vi "AbelFcsMain.vi"() -> ()   [LabVIEW 2011]
uses:
  Camera/vi/ccdChipPixels.vi
  Camera/vi/GlobalSetGetConfigureCamera.vi
  Camera/lib/System Files/user.lib/atmcd32d.llb/Shutter_mode typedef.ctl
  Camera/lib/System Files/user.lib/atmcd32d.llb/Shutter_type typedef.ctl
  Variables/GetPicture.vi
  Camera/vi/StopGetPic.vi
  Camera/vi/CamDef.vi
  Variables/GlobalLaserInterface.vi
  Variables/patternImg.vi
  <vilib>/vision/Image Controls.llb/IMAQ Rounding Mode.ctl
  Variables/GlobalConAxisPI.vi
  Variables/GlobalCameraHandle.vi
  <vilib>/vision/Pattern Matching.llb/IMAQ Match Range Setting.ctl
  <vilib>/vision/Pattern Matching.llb/IMAQ Curve Parameters.ctl
panel:
  out "subarray":dbl[](array[numeric])
  in  "Settings (GeometricMatching)":T3={"Curve Parameters"={"Extraction Mode"=0, "Edge Threshold"=75, "Edge Filter Size"=1, "Min Length"=25, "Row Search Step Size"=15, "Col Search Step Size"=15, "Max Endpoint Gap"=10, "Closed"=FALSE, "Subpixel"=FALSE}, "Match Mode"={"Rotation"=TRUE, "Scale"=FALSE, "Occlusion"=TRUE, "Reserved"=FALSE, "Reserved"=FALSE, "Reserved"=FALSE}, "Range Settings"=[{"Match Constraints"=0, "Min"=0.0, "Max"=360.0}, {"Match Constraints"=2, "Min"=0.0, "Max"=25.0}], "Number of Matches"=5, "Minimum Match Score"=600.0, "SubPixel Accuracy"=FALSE, "Adv. Geometric Match Options 2"=[{"Setup Data Item"=21, "Item Value"=0.0}, {"Setup Data Item"=22, "Item Value"=1.0}]} {"Curve Parameters"."Extraction Mode" items=["Normal", "Uniform Regions"]; "Curve Parameters"."Edge Filter Size" items=["Fine", "Normal", "Contour Tracing"]; "Curve Parameters"."Max Endpoint Gap" min=0; "Curve Parameters"."Col Search Step Size" min=1 max=255 step=1; "Curve Parameters"."Row Search Step Size" min=1 max=255 step=1; "Curve Parameters"."Min Length" min=0; "Curve Parameters"."Edge Threshold" min=1 max=350 step=1; "Range Settings"."Max" format="%.2f"; "Range Settings"."Min" format="%.2f"; "Range Settings"."Match Constraints" items=["Rotation Angle (degrees)", "Scale Factor (%)", "Occlusion (%)"]; "Adv. Geometric Match Options 2"."Setup Data Item" items=["Curve Extraction Mode", "Curve Edge Threshold", "Curve Edge Filter Size", "Min Curve Length", "Curve Row Search Step Size", "Curve Col Search Step Size", "Curve Max Endpoint Gap", "Extract Closed Curves", "Enable Subpixel Curve Extraction", "Enable Correlation Score", "Enable Subpixel Accuracy", "Subpixel Iterations", "Subpixel Tolerance", "Initial Match List Length", "Enable Target Template Curve Score", "Min Match Separation Distance", "Min Match Separation Angle", "Min Match Separation Scale", "Max Match Overlap", "Enable Coarse Result", "Enable Calibration Support", "Enable Contrast Reversal", "Search Strategy", "Refinement Match Factor", "Subpixel Match Factor"]}
  in  "Tab Control":T4(tab)
  out "Histogram":i32[][](graph)
  out "Trace":i32[][](graph)=[[2, 0, 0, 1, 1, 1, 0, 0, 0, 1, 0, 1, 0, 1, 2, 2, 0, 3, 0, 2, 2, 1, 3, 1, 0, 1, 1, 1, 0, 1, 3, 1, 0, 2, 0, 1, 0, 1, 1, 0, 1, 1, 3, 1, 0, 2, 0, 1, 1, 0, 0, 2, 0, 0, 1, 1, 1, 0, 0, 1, 0, 1, 0, 0, 0, 1, 2, 1, 1, 2, 0, 2, 4, 3, 1, 1, 0, 0, 1, 1, 2, 0, 1, 1, 0, 0, 0, 1, 1, 1, 1, 3, 0, 0, 1, 0, 0, 0, 2, 1, 1, 1, 2, 1, 0, 1, 1, 0, 0, 2, 1, 1, 0, 0, 1, 1, 1, 1, 0, 2, 2, 0, 1, 2, 1, 0, 3, 0, 2, 1, 3, 0, 1, 1, 0, 0, 3, 0, 0, 0, 0, 0, 0, 0, 0, 0, 0, 0, 0, 0, 0, 0, 0, 0, 0, 0, 0, 0, 0, 0, 0, 0, 0, 0, 0, 0, 0, 0, 0, 0, 0, 0, 0, 0, 0, 0, 0, 0, 0, 0, 0, 0, 0, 0, 0, 0, 0, 0, 0, 0, 0, 0, 0, 0, 0, 0, 0, 0, 0, 0], [1, 2, 2, 0, 0, 0, 1, 2, 1, 2, 1, 1, 1, 0, 0, 0, 3, 1, 0, 1, 0, 2, 0, 2, 1, 1, 0, 0, 1, 0, 1, 2, 1, 0, 0, 0, 0, 0, 1, 0, 1, 0, 2, 0, 1, 0, 0, 0, 0, 1, 1, 3, 0, 0, 0, 2, 0, 0, 2, 0, 1, 1, 0, 0, 2, 0, 2, 1, 0, 1, 1, 0, 1, 1, 0, 0, 0, 1, 0, 0, 1, 0, 0, 0, 0, 1, 0, 1, 1, 1, 1, 0, 0, 0, 1, 1, 1, 0, 1, 0, 0, 0, 1, 1, 1, 0, 0, 1, 1, 3, 1, 0, 0, 0, 0, 0, 0, 0, 1, 2, 1, 0, 0, 0, 2, 3, 3, 2, 0, 1, 1, 1, 0, 0, 4, 0, 1, 2, 0, 0, 0, 2, 0, 0, 0, 0, 0, 0, 0, 0, 0, 0, 0, 0, 0, 0, 0, 0, 0, 0, 0, 0, 0, 0, 0, 0, 0, 0, 0, 0, 0, 0, 0, 0, 0, 0, 0, 0, 0, 0, 0, 0, 0, 0, 0, 0, 0, 0, 0, 0, 0, 0, 0, 0, 0, 0, 0, 0, 0, 0], [2, 2, 0, 1, 2, 0, 1, 0, 2, 3, 1, 0, 1, 0, 1, 0, 0, 0, 0, 2, 1, 0, 0, 2, 2, 0, 0, 0, 3, 0, 0, 2, 2, 2, 0, 3, 0, 3, 1, 3, 1, 3, 1, 0, 3, 1, 3, 3, 1, 1, 1, 1, 2, 0, 1, 0, 1, 1, 1, 3, 0, 2, 3, 1, 1, 1, 0, 1, 0, 1, 2, 3, 1, 2, 1, 3, 0, 2, 0, 2, 0, 1, 0, 2, 2, 1, 1, 3, 1, 2, 1, 1, 1, 3, 0, 0, 0, 0, 1, 1, 1, 0, 1, 0, 2, 1, 1, 0, 1, 0, 1, 2, 2, 2, 2, 0, 1, 0, 0, 0, 1, 1, 2, 0, 0, 1, 5, 2, 2, 0, 2, 0, 2, 2, 2, 0, 1, 0, 6, 0, 0, 0, 0, 0, 0, 0, 0, 0, 0, 0, 0, 0, 0, 0, 0, 0, 0, 0, 0, 0, 0, 0, 0, 0, 0, 0, 0, 0, 0, 0, 0, 0, 0, 0, 0, 0, 0, 0, 0, 0, 0, 0, 0, 0, 0, 0, 0, 0, 0, 0, 0, 0, 0, 0, 0, 0, 0, 0, 0, 0], [0, 0, 1, 0, 1, 1, 0, 0, 0, 1, 1, 0, 1, 0, 0, 0, 0, 0, 2, 0, 0, 0, 0, 2, 0, 0, 0, 1, 1, 2, 1, 1, 1, 2, 1, 0, 0, 3, 0, 1, 1, 0, 0, 0, 0, 1, 0, 0, 2, 1, 0, 0, 1, 1, 1, 2, 2, 0, 1, 0, 0, 1, 0, 1, 1, 0, 0, 2, 1, 1, 2, 1, 1, 0, 0, 0, 0, 2, 1, 0, 0, 0, 0, 1, 0, 1, 0, 0, 0, 0, 1, 0, 0, 0, 0, 1, 0, 1, 1, 1, 0, 2, 3, 1, 1, 0, 1, 1, 1, 0, 1, 0, 0, 1, 1, 0, 2, 0, 0, 0, 0, 3, 0, 0, 0, 0, 0, 0, 0, 0, 1, 0, 2, 0, 0, 0, 1, 2, 2, 0, 1, 0, 0, 0, 0, 0, 0, 0, 0, 0, 0, 0, 0, 0, 0, 0, 0, 0, 0, 0, 0, 0, 0, 0, 0, 0, 0, 0, 0, 0, 0, 0, 0, 0, 0, 0, 0, 0, 0, 0, 0, 0, 0, 0, 0, 0, 0, 0, 0, 0, 0, 0, 0, 0, 0, 0, 0, 0, 0, 0]]
  out "Point":dbl[][](graph)
  out "Image Out":T5(plugin-control)
  out "Image Number":u32
  out "acquired FPS":dbl
  out "Image":i32[][](graph)
  out "AM image":T5(plugin-control)
  out "Number of Particles":i32
  out "Image 2":dbl[][](graph)
  out "Auto Measure Points":i32
  out "NxtAutMesPoint":i32
  out "Pattern":dbl[][](array[numeric])
  out "X Steps":dbl
  out "3dAbelFcs":bool=TRUE
  out "Y Steps":dbl
  out "Z Steps":dbl
  out "concatenated string":string
  out "Global Stop":bool=TRUE
  out "Stop Measurement":bool
  in  "DeviceTabs":T6(tab)
  in  "WS File Tree":string(tree)
  out "Workspace":path=path "X:/MTusers/Christoph/2011-02-01 Andi/2011-02-01.msw"
  in  "New MSW":bool
  in  "Open MSW":bool
  in  "Sample description":string
  in  "Save Files":bool=TRUE
  out "Last Image File No":i32=-1
  in  "Get Position":bool
  in  "Move Stage":bool
  in  "X-Position":dbl=48.0021 caption="X" min=0.0 max=200.0 step=0.1 format="%1.3f um"
  in  "Y-Position":dbl=19.9997 caption="Y" min=0.0 max=200.0 step=0.1 format="%1.3f um"
  in  "Z-Position":dbl=69.999 caption="Z" min=0.0 max=200.0 step=0.1 format="%1.3f um"
  out "x-position":dbl format="%.3f"
  out "y-position":dbl format="%.3f"
  out "z-position":dbl format="%.3f"
  in  "CFD Settings":T7={"Sync Level"=17, "Sync ZeroX"=0, "Sync Offset"=0, "Chan Settings"=[{"CHx Level"=50, "CHx ZeroX"=10, "CHx Offset"=-22150}, {"CHx Level"=50, "CHx ZeroX"=10, "CHx Offset"=-21850}, {"CHx Level"=75, "CHx ZeroX"=10, "CHx Offset"=-6000}, {"CHx Level"=75, "CHx ZeroX"=10, "CHx Offset"=-5700}]}
  in  "Laser  Profile":string="1"
  in  "Auto Exposure::Mode":u32(ring) items=["Relative"=0, "Ignored"=5]
  in  "Brightness::Mode":u32(ring) items=["Relative"=0, "Ignored"=5]
  in  "Gain::Mode":u32(ring) items=["Absolute"=1, "Auto"=3, "Relative"=0, "Ignored"=5]
  in  "Gamma::Mode":u32(ring)=2 items=["Relative"=0, "Off"=2, "Ignored"=5]
  in  "Shutter::Mode":u32(ring) items=["Auto"=3, "Relative"=0, "Ignored"=5]
  in  "Trigger::Trigger Activation":u32(ring) items=["Level Low", "Level High"]
  in  "Trigger::Trigger Mode":u32(ring)=16 items=["Mode 0"=0, "Mode 1"=1, "Mode 15"=15, "Off"=16]
  in  "Trigger Delay::Mode":u32(ring)=2 items=["Absolute"=1, "Relative"=0, "Off"=2, "Ignored"=5]
  in  "Brightness::Value":dbl=16.0 min=0.0 max=1023.0 step=1.0
  in  "Shutter::Value":dbl=436.0 min=1.0 max=4095.0 step=1.0
  in  "Auto Exposure::Value":dbl=125.0 min=50.0 max=205.0 step=1.0
  in  "Gain::Value":dbl min=0.0 max=680.0 step=1.0
  in  "Trigger::Trigger Parameter":u32 max=0
  in  "Get Temperature":bool
  in  "SET CCD":bool
  in  "OPEN SHUTER":bool
  in  "Close":bool
  in  "Gain":bool
  in  "Start":bool
  in  "Stop":bool
  in  "Exposure":bool
  in  "Set Temperature":bool
  in  "duty cycle":dbl=0.5 format="%.6f"
  in  "frequency":dbl=1.0 format="%.6f"
  in  "PI SystemNumber":i32=1
  in  "Image Measurent Parameters":T8
  in  "Measurement Tab Control":T9(tab)
  in  "SCANNER EMERGENCY":bool
  in  "Stop Program":bool
  out "Task":T10(ring)
  in  "Point Defocussed Cam":bool
  in  "Adjustment":bool
  in  "Laser pulse duration":i32[](array[numeric]) min=2 max=100000 step=1 format="%d µs"
  in  "Measurement Time":i32=60 min=10 format="%.0d s"
  in  "Point Measurement":bool
  out "Counts":u32[](array[numeric])
  in  "Axis":enum32{"x-y", "x-z", "y-x", "y-z", "z-x", "z-y"}(ring)
  in  "Picture size 2":dbl=10.0 min=0.1 max=200.0 format="%1.1f um"
  in  "Picture size":dbl=10.0 min=0.1 max=200.0 format="%1.1f um"
  in  "Pixel time":dbl=3.0 min=0.1 max=100.0 step=0.1 format="%.1f ms"
  in  "Resolution":dbl=0.08 min=0.01 max=10.0 step=0.01 format="%.2f µm"
  out "Measure. time":dbl format="%7.1f s"
  in  "Aquire Image":bool
  out "y":i16=500
  out "x":i16=500
  in  "Save Color Image":bool
  in  "Cam (Defocused)":bool
  in  "How long?":bool
  out "Estimated Time (h)":dbl
  in  "Mesaurement Time (Sec) / Step":dbl
  in  "Start 3D FCS Abel Scan":bool
  in  "FCS Point Measurement":bool
  in  "Z Stepsize":dbl
  in  "Y Stepsize":dbl
  in  "X Stepsize":dbl
  in  "Z End":dbl
  in  "Y End":dbl
  in  "X End":dbl
  in  "Z Start":dbl
  in  "Y Start":dbl
  in  "X Start":dbl
  in  "Find Mols":bool
  in  "Filter":bool=TRUE
  in  "Remove Outliers":i32=10
  in  "Exclude / Include X":bool
  in  "X Start 2":dbl
  in  "X End 2":dbl
  in  "Exclude / Include Y":bool
  in  "Y Start 2":dbl
  in  "Y End 2":dbl
  in  "Measurement Parameter 1":T11 items=["Center of Mass X", "Center of Mass Y", "First Pixel X", "First Pixel Y", "Bounding Rect Left", "Bounding Rect Top", "Bounding Rect Right", "Bounding Rect Bottom", "Max Feret Diameter Start X", "Max Feret Diameter Start Y", "Max Feret Diameter End X", "Max Feret Diameter End Y", "Max Horiz. Segment Length Left", "Max Horiz. Segment Length Right", "Max Horiz. Segment Length Row", "-", "Bounding Rect Width", "Bounding Rect Height", "Bounding Rect Diagonal", "Perimeter", "Convex Hull Perimeter", "Holes' Perimeter", "Max Feret Diameter", "Equivalent Ellipse Major Axis", "Equivalent Ellipse Minor Axis", "Equivalent Ellipse Minor Axis (Feret)", "Equivalent Rect Long Side", "Equivalent Rect Short Side", "Equivalent Rect Diagonal", "Equivalent Rect Short Side (Feret)", "Average Horiz. Segment Length", "Average Vert. Segment Length", "Hydraulic Radius", "Waddel Disk Diameter", "-", "Area", "Holes' Area", "Particle & Holes' Area", "Convex Hull Area", "Image Area", "-", "Number of Holes", "Number of Horiz. Segments", "Number of Vert. Segments", "-", "Orientation", "Max Feret Diameter Orientation", "-", "% Area/Image Area", "% Area/(Particle & Holes' Area)", "Ratio of Equivalent Ellipse Axes", "Ratio of Equivalent Rect Sides", "-", "Elongation Factor", "Compactness Factor", "Heywood Circularity Factor", "Type Factor", "-", "Sum X", "Sum Y", "Sum XX", "Sum XY", "Sum YY", "Sum XXX", "Sum XXY", "Sum XYY", "Sum YYY", "-", "Moment of Inertia XX", "Moment of Inertia XY", "Moment of Inertia YY", "Moment of Inertia XXX", "Moment of Inertia XXY", "Moment of Inertia XYY", "Moment of Inertia YYY", "Norm. Moment of Inertia XX", "Norm. Moment of Inertia XY", "Norm. Moment of Inertia YY", "Norm. Moment of Inertia XXX", "Norm. Moment of Inertia XXY", "Norm. Moment of Inertia XYY", "Norm. Moment of Inertia YYY", "Hu Moment 1", "Hu Moment 2", "Hu Moment 3", "Hu Moment 4", "Hu Moment 5", "Hu Moment 6", "Hu Moment 7"]
  in  "Range Lower Value Par 1":dbl
  in  "Range Upper Value  Par 1":dbl
  in  "Ex/In Par 1":bool
  in  "Measurement Parameter 2":T11 items=["Center of Mass X", "Center of Mass Y", "First Pixel X", "First Pixel Y", "Bounding Rect Left", "Bounding Rect Top", "Bounding Rect Right", "Bounding Rect Bottom", "Max Feret Diameter Start X", "Max Feret Diameter Start Y", "Max Feret Diameter End X", "Max Feret Diameter End Y", "Max Horiz. Segment Length Left", "Max Horiz. Segment Length Right", "Max Horiz. Segment Length Row", "-", "Bounding Rect Width", "Bounding Rect Height", "Bounding Rect Diagonal", "Perimeter", "Convex Hull Perimeter", "Holes' Perimeter", "Max Feret Diameter", "Equivalent Ellipse Major Axis", "Equivalent Ellipse Minor Axis", "Equivalent Ellipse Minor Axis (Feret)", "Equivalent Rect Long Side", "Equivalent Rect Short Side", "Equivalent Rect Diagonal", "Equivalent Rect Short Side (Feret)", "Average Horiz. Segment Length", "Average Vert. Segment Length", "Hydraulic Radius", "Waddel Disk Diameter", "-", "Area", "Holes' Area", "Particle & Holes' Area", "Convex Hull Area", "Image Area", "-", "Number of Holes", "Number of Horiz. Segments", "Number of Vert. Segments", "-", "Orientation", "Max Feret Diameter Orientation", "-", "% Area/Image Area", "% Area/(Particle & Holes' Area)", "Ratio of Equivalent Ellipse Axes", "Ratio of Equivalent Rect Sides", "-", "Elongation Factor", "Compactness Factor", "Heywood Circularity Factor", "Type Factor", "-", "Sum X", "Sum Y", "Sum XX", "Sum XY", "Sum YY", "Sum XXX", "Sum XXY", "Sum XYY", "Sum YYY", "-", "Moment of Inertia XX", "Moment of Inertia XY", "Moment of Inertia YY", "Moment of Inertia XXX", "Moment of Inertia XXY", "Moment of Inertia XYY", "Moment of Inertia YYY", "Norm. Moment of Inertia XX", "Norm. Moment of Inertia XY", "Norm. Moment of Inertia YY", "Norm. Moment of Inertia XXX", "Norm. Moment of Inertia XXY", "Norm. Moment of Inertia XYY", "Norm. Moment of Inertia YYY", "Hu Moment 1", "Hu Moment 2", "Hu Moment 3", "Hu Moment 4", "Hu Moment 5", "Hu Moment 6", "Hu Moment 7"]
  in  "Range Lower Value Par 2":dbl
  in  "Range Upper Value Par 2":dbl
  in  "Ex/In Par 2":bool
  in  "Square/Hexa":bool=TRUE
  in  "Connectivity 4/8":bool
  in  "Manual":bool
  in  "Focuswidth":dbl
  in  "Mode":enum16{"Gauss", "Radial", "Azimuthal"}(ring)
  in  "Detection Modus":u16(ring) items=["Pattern", "Heuristic"]
  in  "NA":dbl
  in  "TSH":dbl min=0.0 max=1.0 step=0.01
  in  "Auto Defocussed Cam":bool
  in  "Autopoint-Autofocus Z":bool=TRUE
  in  "Auto Measurement Time (ms)":i32=60 caption="Measurement Time (s)" min=10
  out "Auto Meas Progress":i32(slide) caption="Point 34 / 34" scale=0.0..34.0
  in  "Auto Meas":bool
  out "Active pt3":path
  out "Buffer Overrun":bool
  out "Running":bool
  # "Range"
  # "Scanner Position"
  # "Point Measurement Settings"
  # "Start Experiment"
  # "Estimated Mesaurement Time"
  # "Image Scan Settings"
  # "Save as png"
  # "Pixel"
  # "Define the 3D Space and Stepwith of your Experiment"
  # "Time of the Experiment"
  # "Check What to Mesaure"
  # "Start Your Experiment here"
  # "Lifetime Mesaurement Time on each Position"
  # "Define Search Area"
  # "Define Detection Parameters"
  # "Exact Matching"
  # "Operation"
  # "Show Progress"
  # "Automated Mesaurement on Single Molecule Coordinates on the  2D Frame"
  # "Start Your Experiment here"
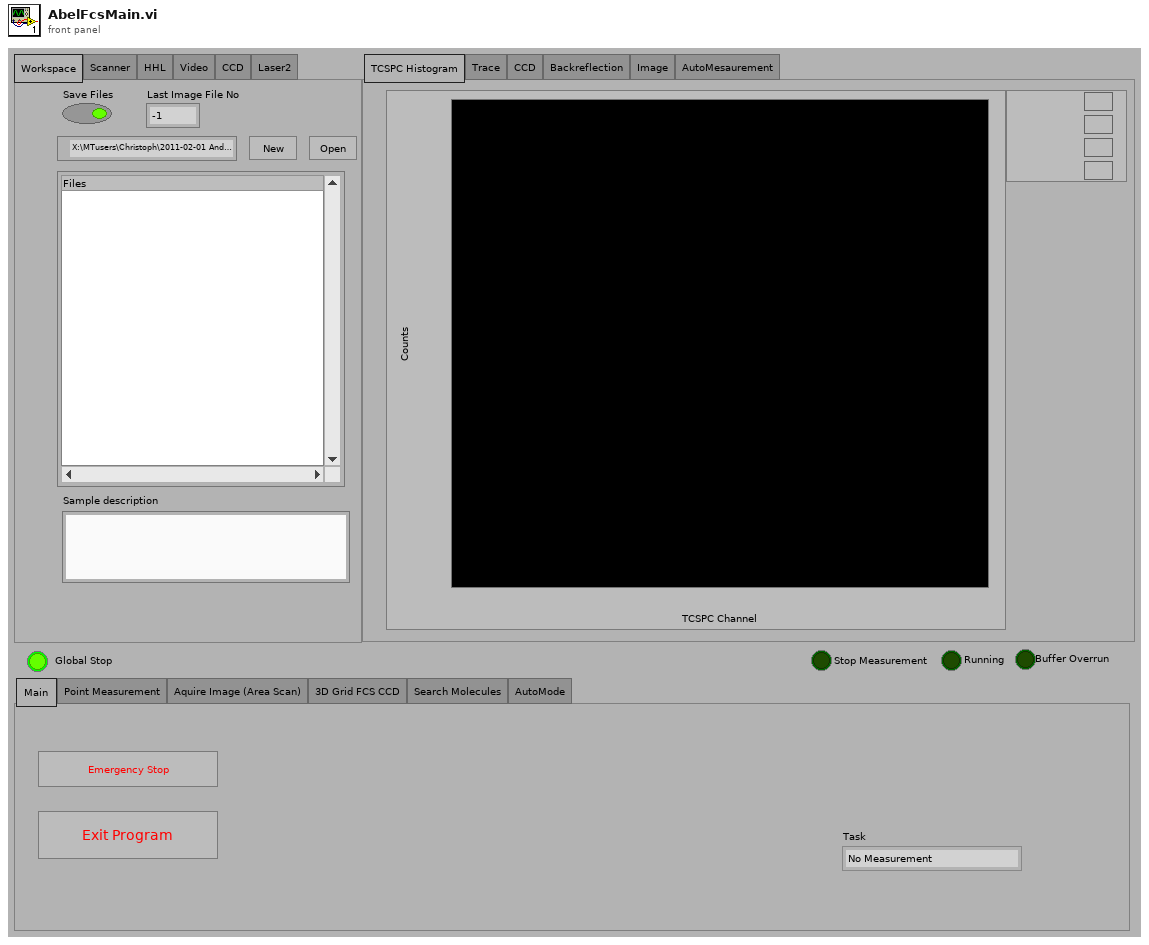
[diagram p1: front panel]
types:
  T1 = typedef "IMAQ Curve Parameters.ctl" = cluster{"Extraction Mode":u32, "Edge Threshold":i32, "Edge Filter Size":u32, "Min Length":i32, "Row Search Step Size":i32, "Col Search Step Size":i32, "Max Endpoint Gap":i32, "Closed":bool, "Subpixel":bool}
  T2 = typedef "IMAQ Match Range Setting.ctl" = cluster{"Match Constraints":u32, "Min":dbl, "Max":dbl}
  T3 = cluster{"Curve Parameters":T1, "Match Mode":cluster{"Rotation":bool, "Scale":bool, "Occlusion":bool, "Reserved":bool, "Reserved":bool, "Reserved":bool}, "Range Settings":T2[], "Number of Matches":i32, "Minimum Match Score":sgl, "SubPixel Accuracy":bool, "Adv. Geometric Match Options 2":cluster{"Setup Data Item":u16, "Item Value":dbl}[]}
  T4 = enum32{"TCSPC Histogram", "Trace", "CCD", "Backreflection", "Image", "AutoMesaurement"}
  T5 = typedef "IMAQ Image.ctl" = refnum<image>
  T6 = enum32{"Workspace", "Scanner", "HHL", "Video", "CCD", "Laser2"}
  T7 = cluster{"Sync Level":i32, "Sync ZeroX":i32, "Sync Offset":i32, "Chan Settings":cluster{"CHx Level":i32, "CHx ZeroX":i32, "CHx Offset":i32}[]}
  T8 = cluster{"Position":cluster{"X-Position":dbl, "Y-Position":dbl, "Z-Position":dbl}, "Axis 1 Pixels":dbl, "Axis 2 Pixels":dbl, "Axis":i32, "Resolution":dbl, "PixelTime":dbl, "Laser pulses":i32}
  T9 = enum32{"Main ", "Point Measurement", "Aquire Image (Area Scan)", "3D Grid FCS CCD", "Search Molecules", "AutoMode"}
  T10 = enum16{"No Measurement", "Aquire Image", "Point Measurement", "Multi Measurement", "Save Color Image", "Find Single Mol.", "Auto Measurement Control", "Auto Point", "Aquire Line Scan", "Grid Measurement", "Trapping", "Move Scanner"}
  T11 = typedef "Particle Parameters" = i32
  T12 = cluster{"Dev":i32, "SerNo":string, "HW_Model":string, "HW_Partno":string}[]
  T13 = enum16{"No Measurement", "Aquire Image", "Point Measurement", "Multi Measurement", "Save Color Image"}
  T14 = enum16{"No Measurement", "Aquire Image", "Point Measurement", "Multi Measurement", "Save Color Image", "Find Single Mol.", "Auto Measurement Control", "Auto Point"}
  T15 = enum16{"No Measurement", "Aquire Image", "Point Measurement", "Multi Measurement", "Save Color Image", "Find Single Mol."}
  T16 = enum16{"Get (Default)", "Set Workspace", "Append File", "Change Comment"}
  T17 = typedef "Shutter_type typedef.ctl" = enum16{"TTL Low", "TTL High"}
  T18 = typedef "Shutter_mode typedef.ctl" = enum16{"Auto", "Open", "Close"}
  T19 = cluster{"File No":i32, "File Path":path, "Parent File":i32, "File Type":enum16{"unknown", "pt3 File", "png Image", "bmp Image"}, "Measurement Type":enum16{"not a pt3 File", "Image File", "Point Measurement", "Auto Point", "Line Scan", "Grid Scan"}, "Upper Left":cluster{"x-Position":dbl, "y-Position":dbl, "z-Position":dbl}, "Pixels":dbl[], "Resolution":dbl, "Scan Axis":enum32{"x-y", "x-z", "y-x", "y-z", "z-x", "z-y"}, "PixelTime":dbl}[]
  T20 = cluster{"File No":i32, "File Path":path, "Parent File":i32, "File Type":enum16{"unknown", "pt3 File", "png Image", "bmp Image"}, "Measurement Type":enum16{"not a pt3 File", "Image File", "Point Measurement", "Auto Point", "Line Scan", "Grid Scan"}, "Upper Left":cluster{"x-Position":dbl, "y-Position":dbl, "z-Position":dbl}, "Pixels":i32[], "Scan Axis":enum32{"x-y", "x-z", "y-x", "y-z", "z-x", "z-y"}, "Resolution":dbl, "PixelTime":dbl}[]
  T21 = cluster{"File No":i32, "File Path":path, "Parent File":i32, "File Type":enum16{"unknown", "pt3 File", "png Image", "bmp Image"}, "Measurement Type":enum16{"not a pt3 File", "Image File", "Point Measurement", "Auto Point", "Line Scan", "Grid Scan"}, "Upper Left":cluster{"x-Position":dbl, "y-Position":dbl, "z-Position":dbl}, "Pixels":i32[], "Resolution":dbl, "Scan Axis":enum32{"x-y", "x-z", "y-z"}, "PixelTime":dbl}[]
  T22 = cluster{"Files in Workspace[0]":cluster{"File No":i32, "File Path":path, "Parent File":i32, "File Type":enum16{"unknown", "pt3 File", "png Image", "bmp Image"}, "Measurement Type":enum16{"not a pt3 File", "Image File", "Point Measurement", "Auto Point", "Line Scan", "Grid Scan"}, "Upper Left":cluster{"x-Position":dbl, "y-Position":dbl, "z-Position":dbl}, "Pixels":i32[], "Scan Axis":enum32{"x-y", "x-z", "y-x", "y-z", "z-x", "z-y"}, "Resolution":dbl, "PixelTime":dbl}, "Files in Workspace[1]":cluster{"File No":i32, "File Path":path, "Parent File":i32, "File Type":enum16{"unknown", "pt3 File", "png Image", "bmp Image"}, "Measurement Type":enum16{"not a pt3 File", "Image File", "Point Measurement", "Auto Point", "Line Scan", "Grid Scan"}, "Upper Left":cluster{"x-Position":dbl, "y-Position":dbl, "z-Position":dbl}, "Pixels":i32[], "Scan Axis":enum32{"x-y", "x-z", "y-x", "y-z", "z-x", "z-y"}, "Resolution":dbl, "PixelTime":dbl}, "Files in Workspace[2]":cluster{"File No":i32, "File Path":path, "Parent File":i32, "File Type":enum16{"unknown", "pt3 File", "png Image", "bmp Image"}, "Measurement Type":enum16{"not a pt3 File", "Image File", "Point Measurement", "Auto Point", "Line Scan", "Grid Scan"}, "Upper Left":cluster{"x-Position":dbl, "y-Position":dbl, "z-Position":dbl}, "Pixels":i32[], "Scan Axis":enum32{"x-y", "x-z", "y-x", "y-z", "z-x", "z-y"}, "Resolution":dbl, "PixelTime":dbl}, "Files in Workspace[3]":cluster{"File No":i32, "File Path":path, "Parent File":i32, "File Type":enum16{"unknown", "pt3 File", "png Image", "bmp Image"}, "Measurement Type":enum16{"not a pt3 File", "Image File", "Point Measurement", "Auto Point", "Line Scan", "Grid Scan"}, "Upper Left":cluster{"x-Position":dbl, "y-Position":dbl, "z-Position":dbl}, "Pixels":i32[], "Scan Axis":enum32{"x-y", "x-z", "y-x", "y-z", "z-x", "z-y"}, "Resolution":dbl, "PixelTime":dbl}, "Files in Workspace[4]":cluster{"File No":i32, "File Path":path, "Parent File":i32, "File Type":enum16{"unknown", "pt3 File", "png Image", "bmp Image"}, "Measurement Type":enum16{"not a pt3 File", "Image File", "Point Measurement", "Auto Point", "Line Scan", "Grid Scan"}, "Upper Left":cluster{"x-Position":dbl, "y-Position":dbl, "z-Position":dbl}, "Pixels":i32[], "Scan Axis":enum32{"x-y", "x-z", "y-x", "y-z", "z-x", "z-y"}, "Resolution":dbl, "PixelTime":dbl}, "Files in Workspace[5]":cluster{"File No":i32, "File Path":path, "Parent File":i32, "File Type":enum16{"unknown", "pt3 File", "png Image", "bmp Image"}, "Measurement Type":enum16{"not a pt3 File", "Image File", "Point Measurement", "Auto Point", "Line Scan", "Grid Scan"}, "Upper Left":cluster{"x-Position":dbl, "y-Position":dbl, "z-Position":dbl}, "Pixels":i32[], "Scan Axis":enum32{"x-y", "x-z", "y-x", "y-z", "z-x", "z-y"}, "Resolution":dbl, "PixelTime":dbl}, "Files in Workspace[6]":cluster{"File No":i32, "File Path":path, "Parent File":i32, "File Type":enum16{"unknown", "pt3 File", "png Image", "bmp Image"}, "Measurement Type":enum16{"not a pt3 File", "Image File", "Point Measurement", "Auto Point", "Line Scan", "Grid Scan"}, "Upper Left":cluster{"x-Position":dbl, "y-Position":dbl, "z-Position":dbl}, "Pixels":i32[], "Scan Axis":enum32{"x-y", "x-z", "y-x", "y-z", "z-x", "z-y"}, "Resolution":dbl, "PixelTime":dbl}, "Files in Workspace[7]":cluster{"File No":i32, "File Path":path, "Parent File":i32, "File Type":enum16{"unknown", "pt3 File", "png Image", "bmp Image"}, "Measurement Type":enum16{"not a pt3 File", "Image File", "Point Measurement", "Auto Point", "Line Scan", "Grid Scan"}, "Upper Left":cluster{"x-Position":dbl, "y-Position":dbl, "z-Position":dbl}, "Pixels":i32[], "Scan Axis":enum32{"x-y", "x-z", "y-x", "y-z", "z-x", "z-y"}, "Resolution":dbl, "PixelTime":dbl}, "Files in Workspace[8]":cluster{"File No":i32, "File Path":path, "Parent File":i32, "File Type":enum16{"unknown", "pt3 File", "png Image", "bmp Image"}, "Measurement Type":enum16{"not a pt3 File", "Image File", "Point Measurement", "Auto Point", "Line Scan", "Grid Scan"}, "Upper Left":cluster{"x-Position":dbl, "y-Position":dbl, "z-Position":dbl}, "Pixels":i32[], "Scan Axis":enum32{"x-y", "x-z", "y-x", "y-z", "z-x", "z-y"}, "Resolution":dbl, "PixelTime":dbl}}
  T23 = typedef "LVPoint32TypeDef.ctl" = cluster{"Horizontal":i32, "Vertical":i32}
  T24 = cluster{"Shift":bool, "Ctrl":bool, "Alt":bool, "Cmd":bool, "Opt":bool}
  T25 = enum16{"No Measurement", "Aquire Image", "Point Measurement", "Multi Measurement", "Save Color Image", "Find Single Mol.", "Auto Measurement Control", "Auto Point", "Aquire Line Scan", "Grid Measurement"}
  T26 = enum16{"none", "fast axis", "slow axis", "both axis", ""}
  T27 = enum16{"none", "fast axis", "slow axis", "both", ""}
  T28 = enum16{"target position", "relative position", "actual position", "position error"}
  T29 = enum16{"not a pt3 File", "Image File", "Point Measurement", "Auto Point"}
  T30 = enum16{"unknown", "pt3 File", "png Image", "bmp Image"}
  T31 = typedef "IMAQ Rounding Mode.ctl" = enum16{"Optimize", "Truncate"}
  T32 = cluster{"Measurement Parameter":T11, "Range Lower Value":dbl, "Range Upper Value":dbl, "Range":bool, "Measurement Type":bool}[]
  T33 = enum16{"not a pt3 File", "Image File", "Point Measurement", "Auto Point", "Line Scan"}
  T34 = cluster{"Dev":i32, "SerNo":string, "HW_Model":string, "HW_Partno":string}
  T35 = cluster{"Comment":string, "Binning":i32, "Offset":i32, "AcquisitionTime (ms)":i32, "HardwareSerial":i32, "SyncDivider":i32, "Resolution (ps)":dbl, "CFD Settings":cluster{"Sync Level":i32, "Sync ZeroX":i32, "Sync Offset":i32, "Chan Settings":cluster{"CHx Level":i32, "CHx ZeroX":i32, "CHx Offset":i32}[]}, "ModuleInfo":cluster{"modelcode":i32, "versioncode":i32}[], "BaseResolution (ps)":dbl, "RefClockSource":i32, "ChanInfo":cluster{"CHx Level":i32, "CHx ZeroX":i32, "CHx Offset":i32, "CHx modidx":i32}[], "SyncRate":i32, "InputsEnabled":i64}
  T36 = cluster{"Dimensions":i32, "Time Per Pixel [ms]":dbl, "Acceleration":i32, "Pattern":i32, "X0":sgl, "Y0":sgl, "Z0":dbl, "PixX":i32, "PixY":i32, "PixResol":sgl, "TStartTo":sgl, "TStoptTo":sgl, "TStartFro":sgl, "TStopFro":sgl}
  T37 = cluster{"InpRateFilePos":i64, "StopAfterFilePos":i64}
  T38 = cluster{"X-Position":dbl, "Y-Position":dbl, "Z-Position":dbl}
  T39 = cluster{"File No":i32, "File Path":path, "Parent File":i32, "File Type":enum16{"unknown", "pt3 File", "png Image", "bmp Image"}, "Measurement Type":enum16{"not a pt3 File", "Image File", "Point Measurement", "Auto Point", "Line Scan", "Grid Scan"}, "Upper Left":cluster{"x-Position":dbl, "y-Position":dbl, "z-Position":dbl}, "Pixels":i32[], "Scan Axis":enum32{"x-y", "x-z", "y-z"}, "Resolution":dbl, "PixelTime":dbl}
  T40 = enum16{"not a pt3 File", "Image File", "Point Measurement", "Auto Point", "Line Scan", "Grid Scan"}
  T41 = cluster{"Ident":string, "Format Version":string, "Creator Name":string, "Creator Version":string, "File Time":string, "Comment":string, "Laser":i32, "Binning":i32, "Offset":i32, "AcquisitionTime (ms)":i32, "HardwareSerial":i32, "SyncDivider":i32, "Resolution (ps)":dbl, "Rates":dbl[], "SyncRate":dbl, "CFD Settings":cluster{"Sync Level":i32, "Sync ZeroX":i32, "Sync Offset":i32, "Chan Settings":cluster{"CHx Level":i32, "CHx ZeroX":i32, "CHx Offset":i32}[]}}
  T42 = cluster{"x-Position":dbl, "y-Position":dbl, "z-Position":dbl}
  T43 = typedef "Image Type" = u32
  T44 = cluster{"MesaurementSelection[0]":cluster{"Measurement Parameter":T11, "Range Lower Value":dbl, "Range Upper Value":dbl, "Range":bool, "Measurement Type":bool}, "MesaurementSelection[1]":cluster{"Measurement Parameter":T11, "Range Lower Value":dbl, "Range Upper Value":dbl, "Range":bool, "Measurement Type":bool}, "MesaurementSelection[2]":cluster{"Measurement Parameter":T11, "Range Lower Value":dbl, "Range Upper Value":dbl, "Range":bool, "Measurement Type":bool}, "MesaurementSelection[3]":cluster{"Measurement Parameter":T11, "Range Lower Value":dbl, "Range Upper Value":dbl, "Range":bool, "Measurement Type":bool}, "MesaurementSelection[4]":cluster{"Measurement Parameter":T11, "Range Lower Value":dbl, "Range Upper Value":dbl, "Range":bool, "Measurement Type":bool}, "MesaurementSelection[5]":cluster{"Measurement Parameter":T11, "Range Lower Value":dbl, "Range Upper Value":dbl, "Range":bool, "Measurement Type":bool}, "MesaurementSelection[6]":cluster{"Measurement Parameter":T11, "Range Lower Value":dbl, "Range Upper Value":dbl, "Range":bool, "Measurement Type":bool}, "MesaurementSelection[7]":cluster{"Measurement Parameter":T11, "Range Lower Value":dbl, "Range Upper Value":dbl, "Range":bool, "Measurement Type":bool}, "MesaurementSelection[8]":cluster{"Measurement Parameter":T11, "Range Lower Value":dbl, "Range Upper Value":dbl, "Range":bool, "Measurement Type":bool}}
  T45 = cluster{"Measurement Parameter":T11, "Range Lower Value":dbl, "Range Upper Value":dbl, "Range":bool, "Measurement Type":bool}
  T46 = typedef "IMAQ Point" = cluster{"X":sgl, "Y":sgl}
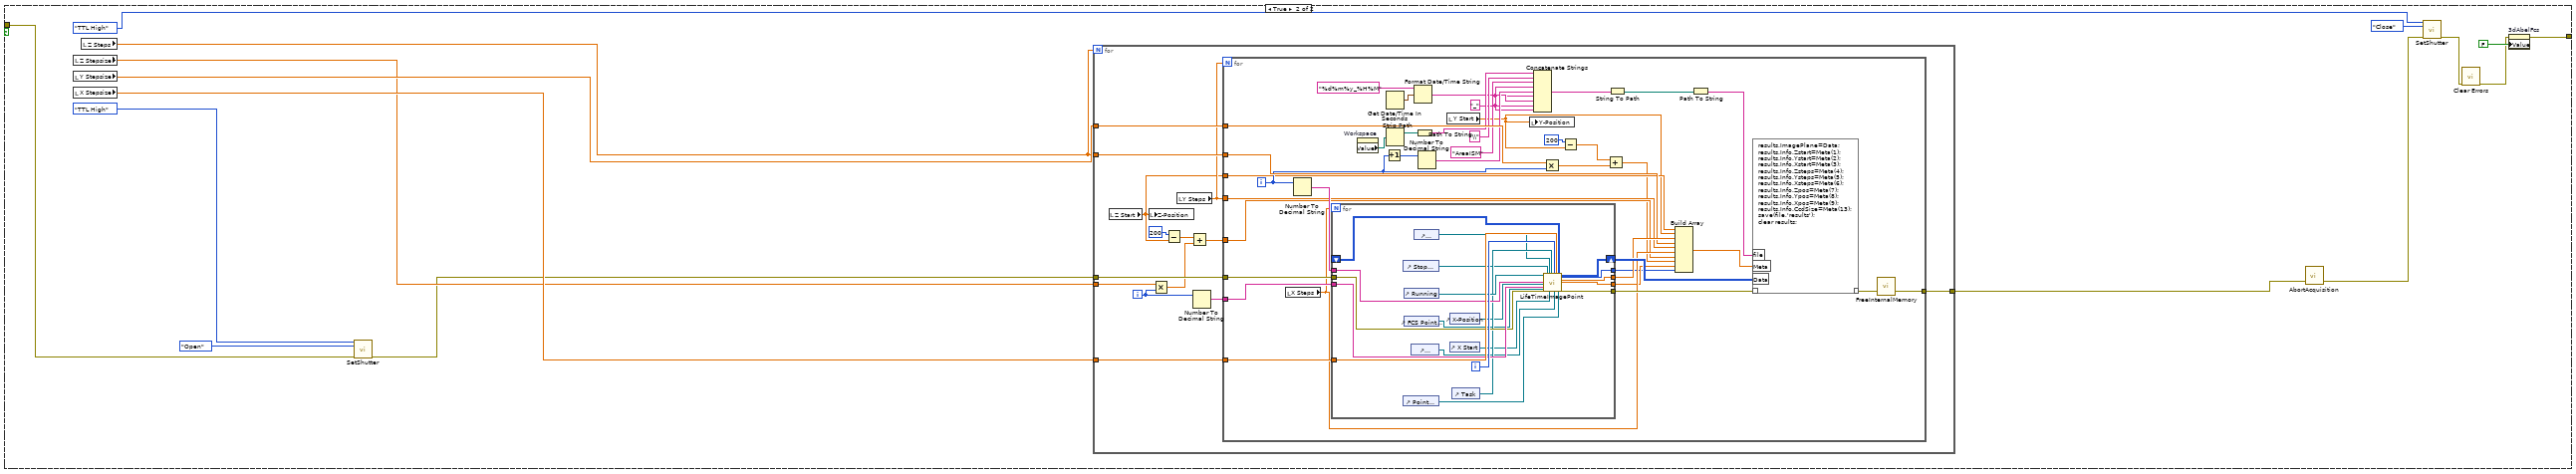
[diagram p2: hidden frame]
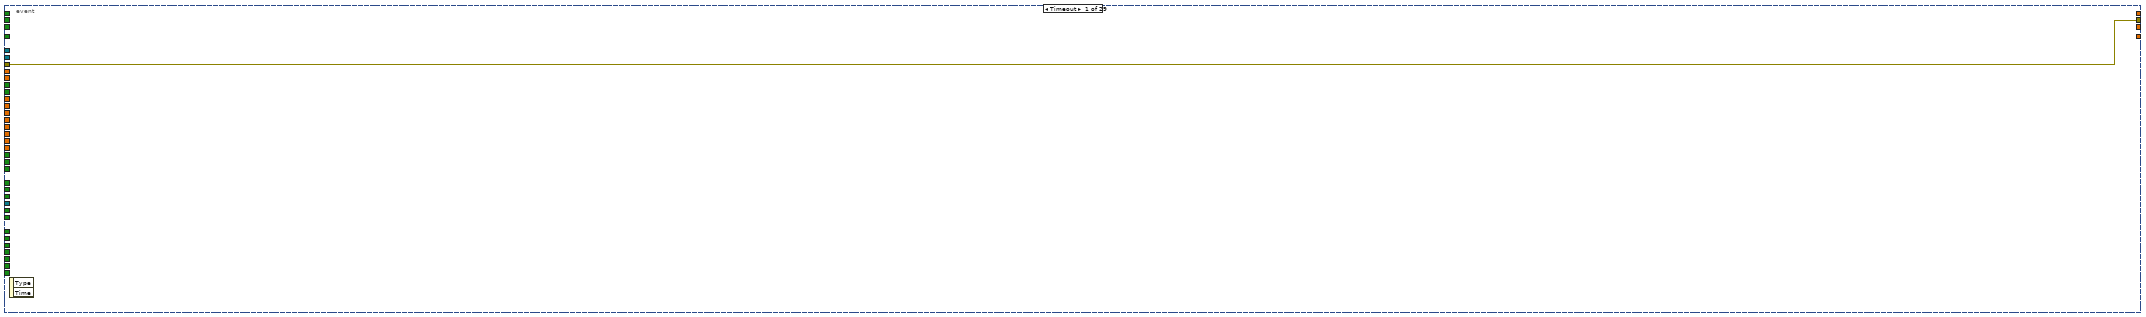
[diagram p3: hidden frame]
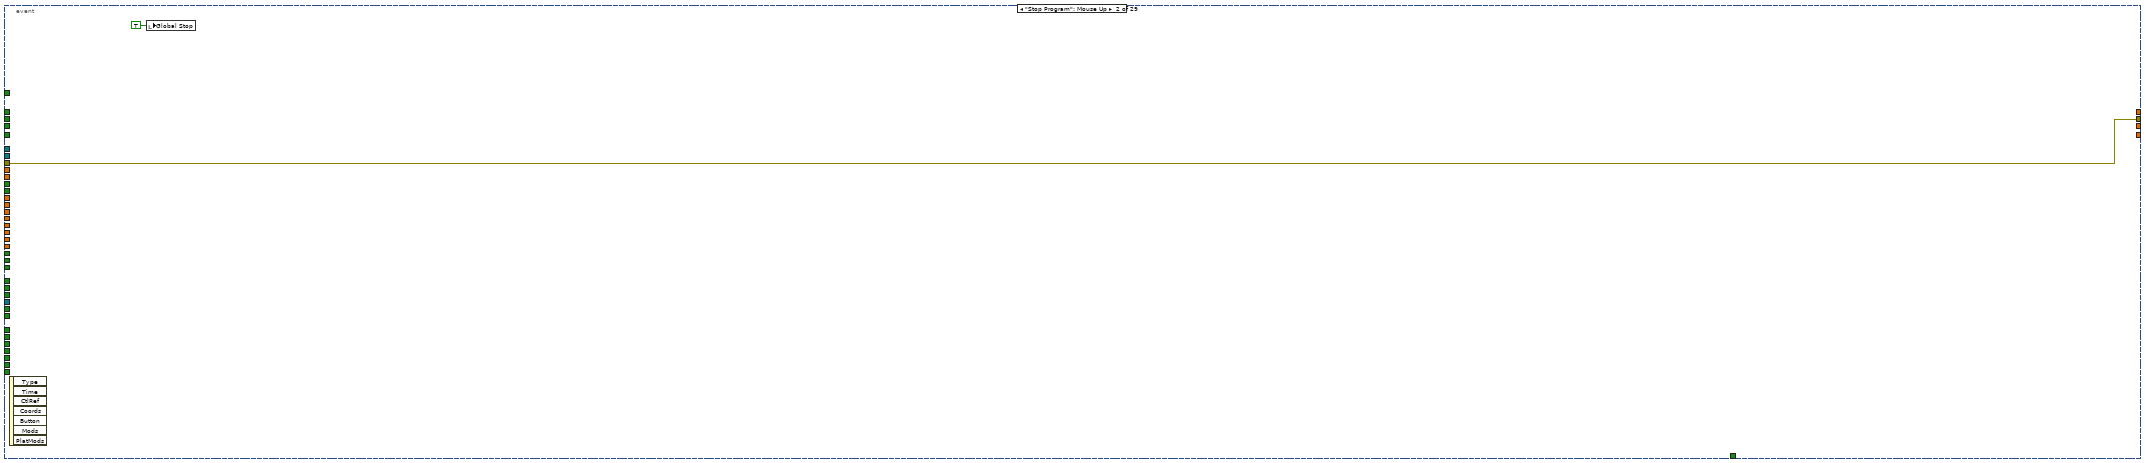
[diagram p4: hidden frame]
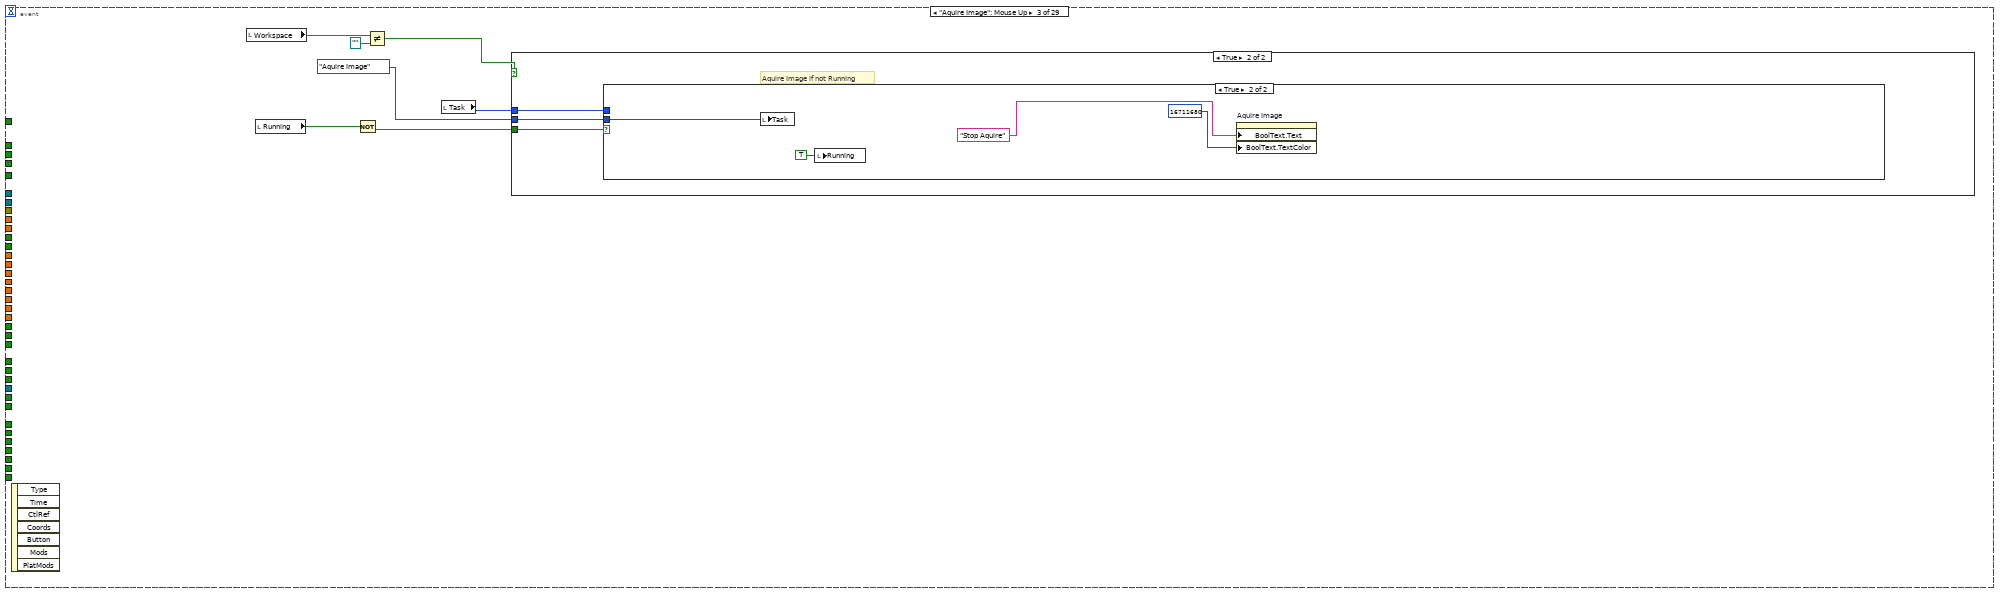
[diagram p5: hidden frame]
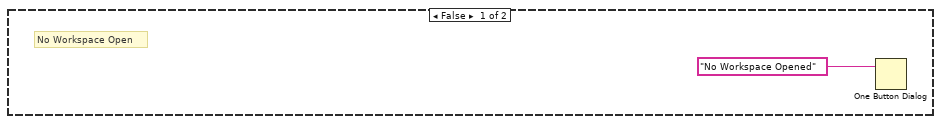
[diagram p6: hidden frame]
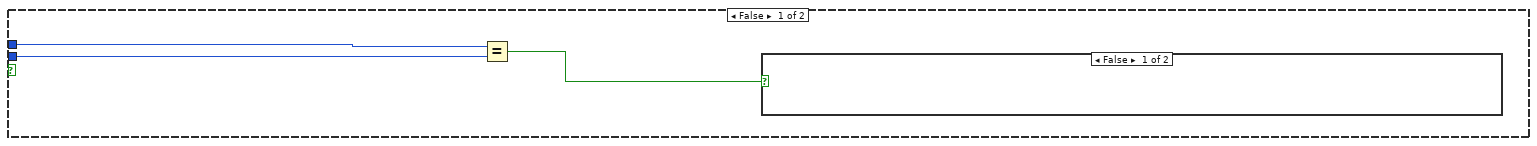
[diagram p7: hidden frame]
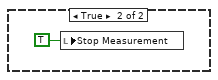
[diagram p8: hidden frame]
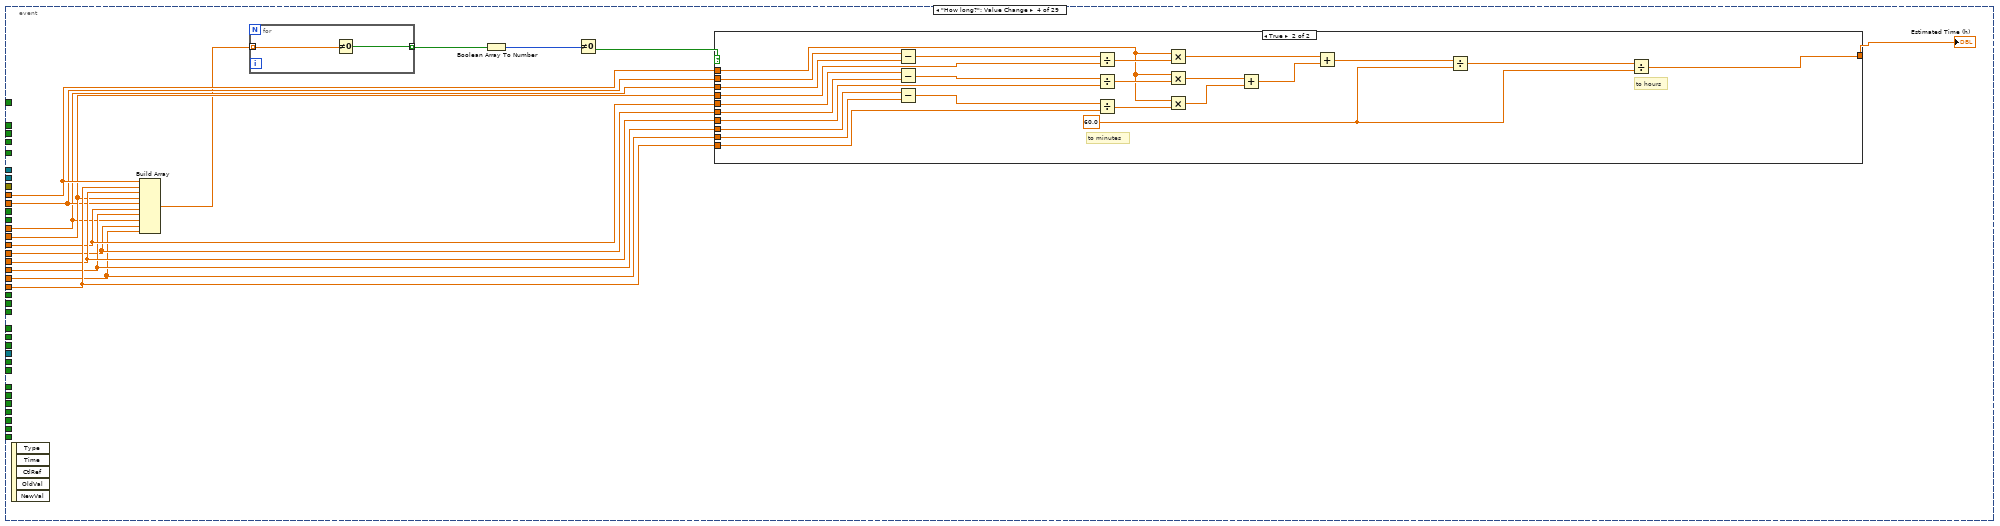
[diagram p9: hidden frame]
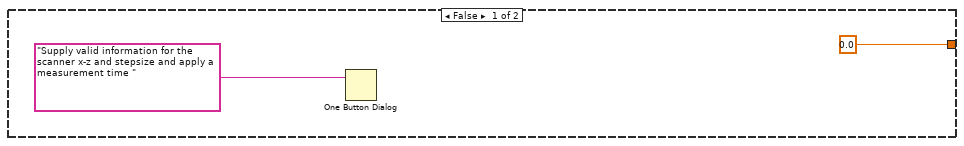
[diagram p10: hidden frame]
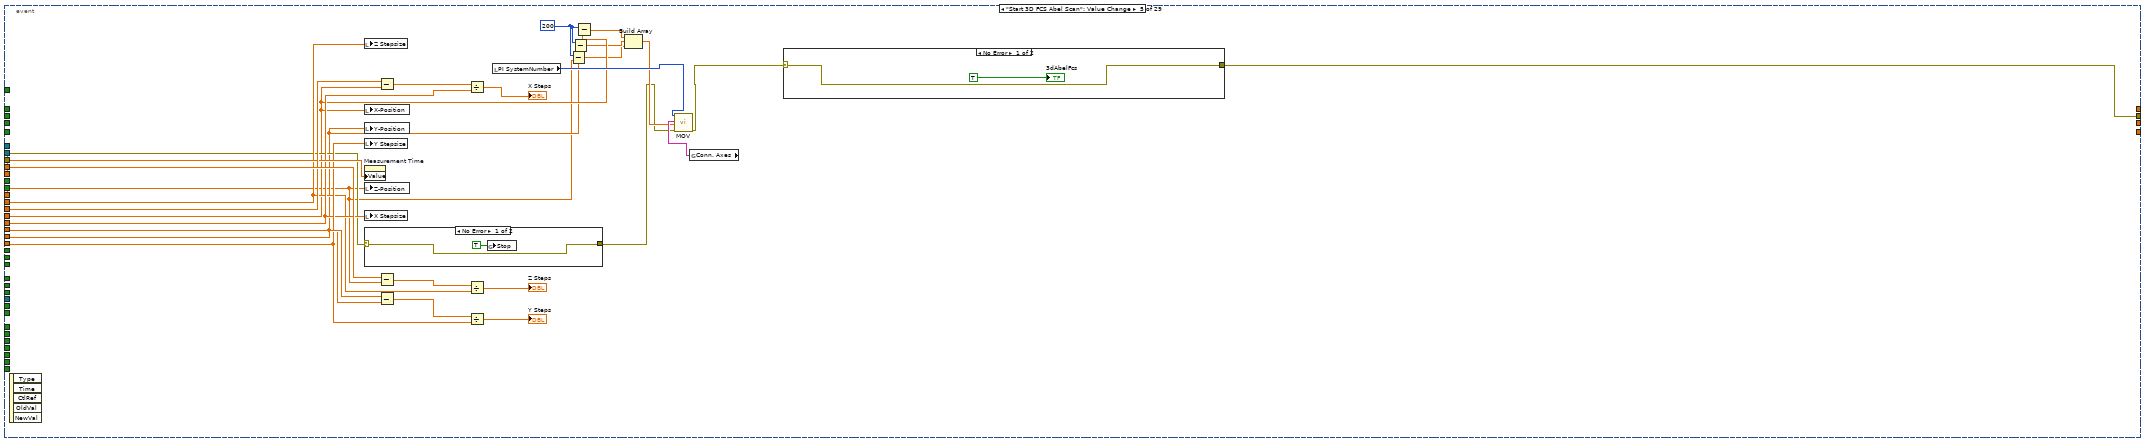
[diagram p11: hidden frame]
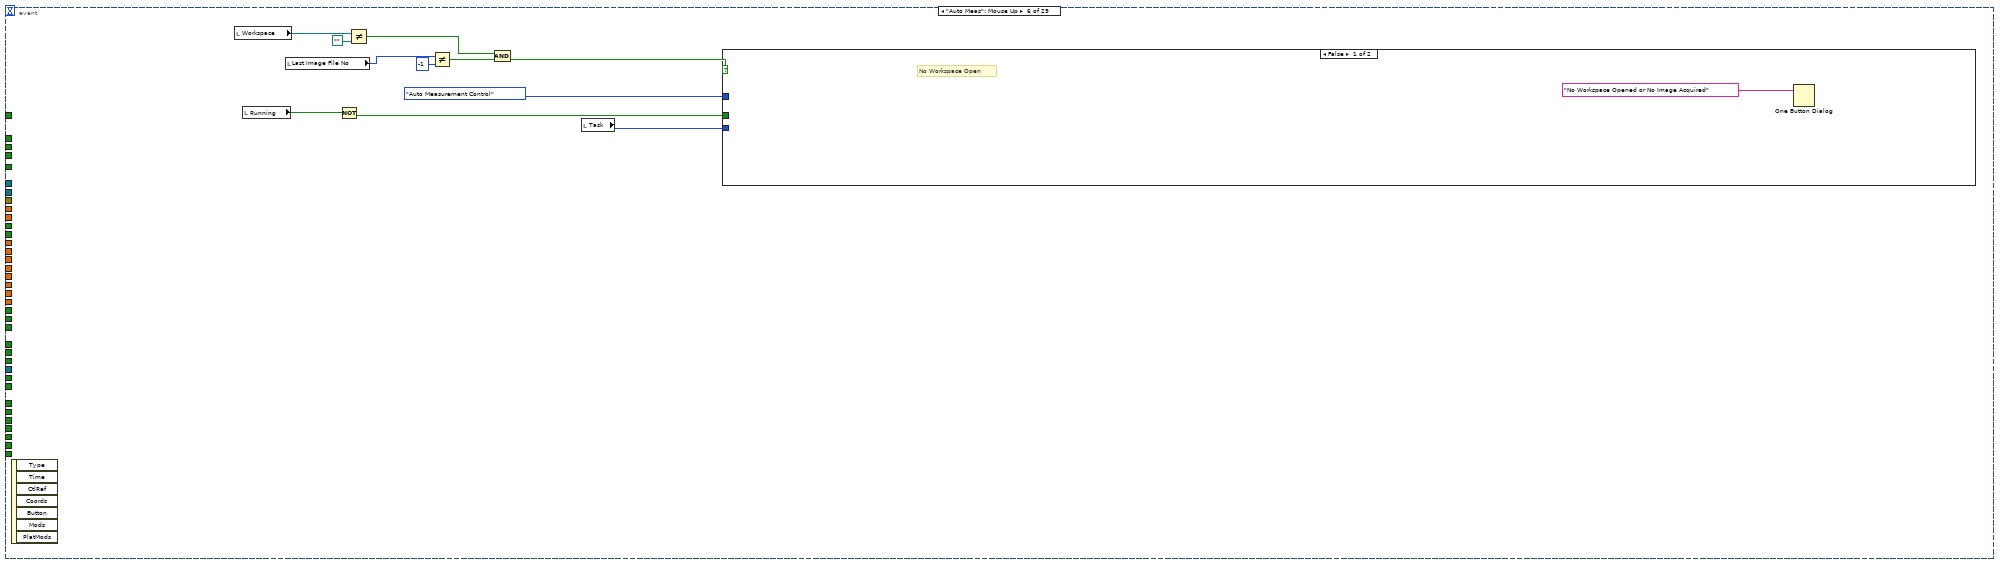
[diagram p14: hidden frame]
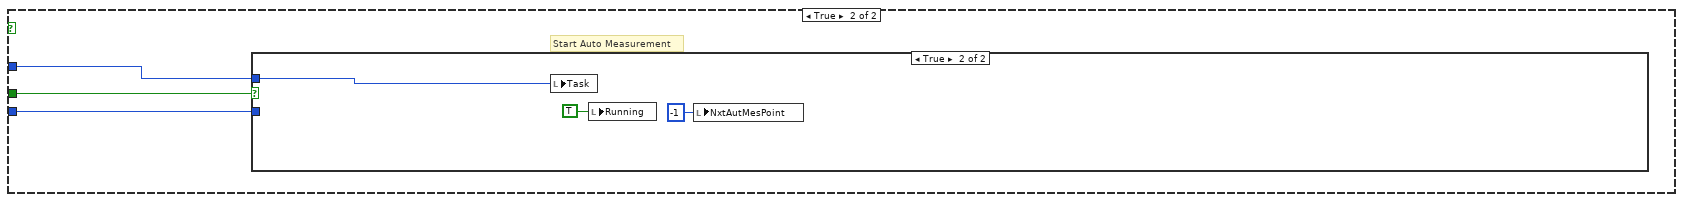
[diagram p15: hidden frame]
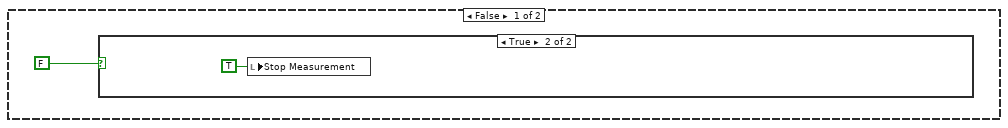
[diagram p16: hidden frame]
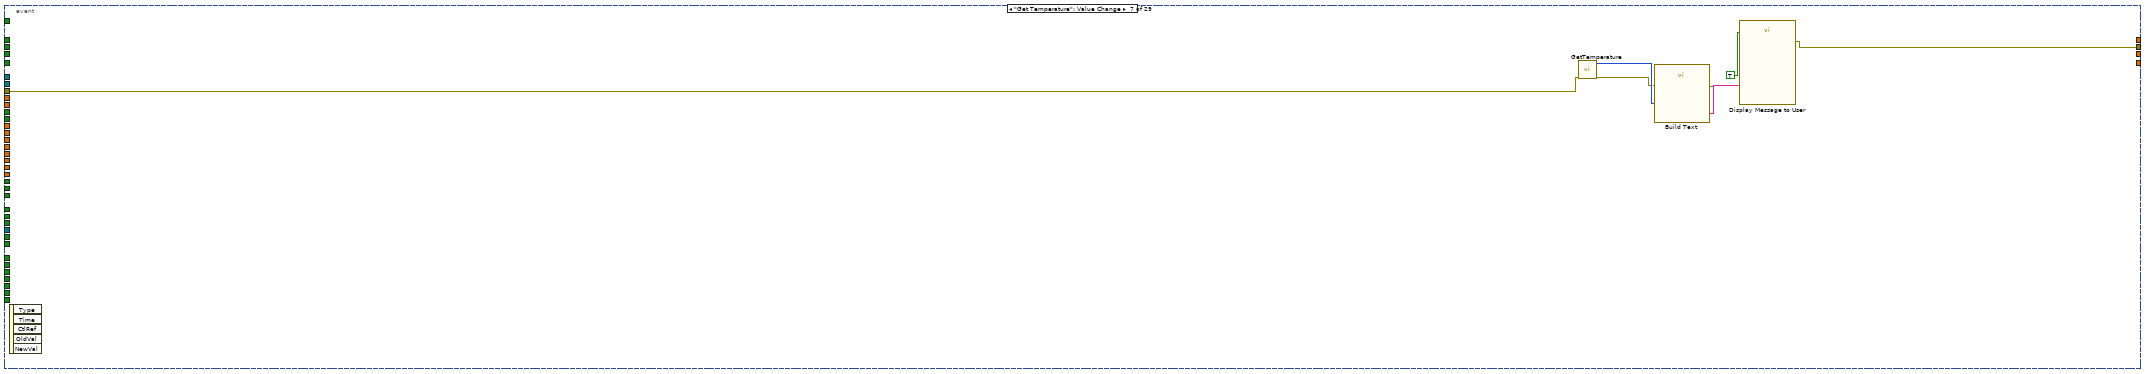
[diagram p18: hidden frame]
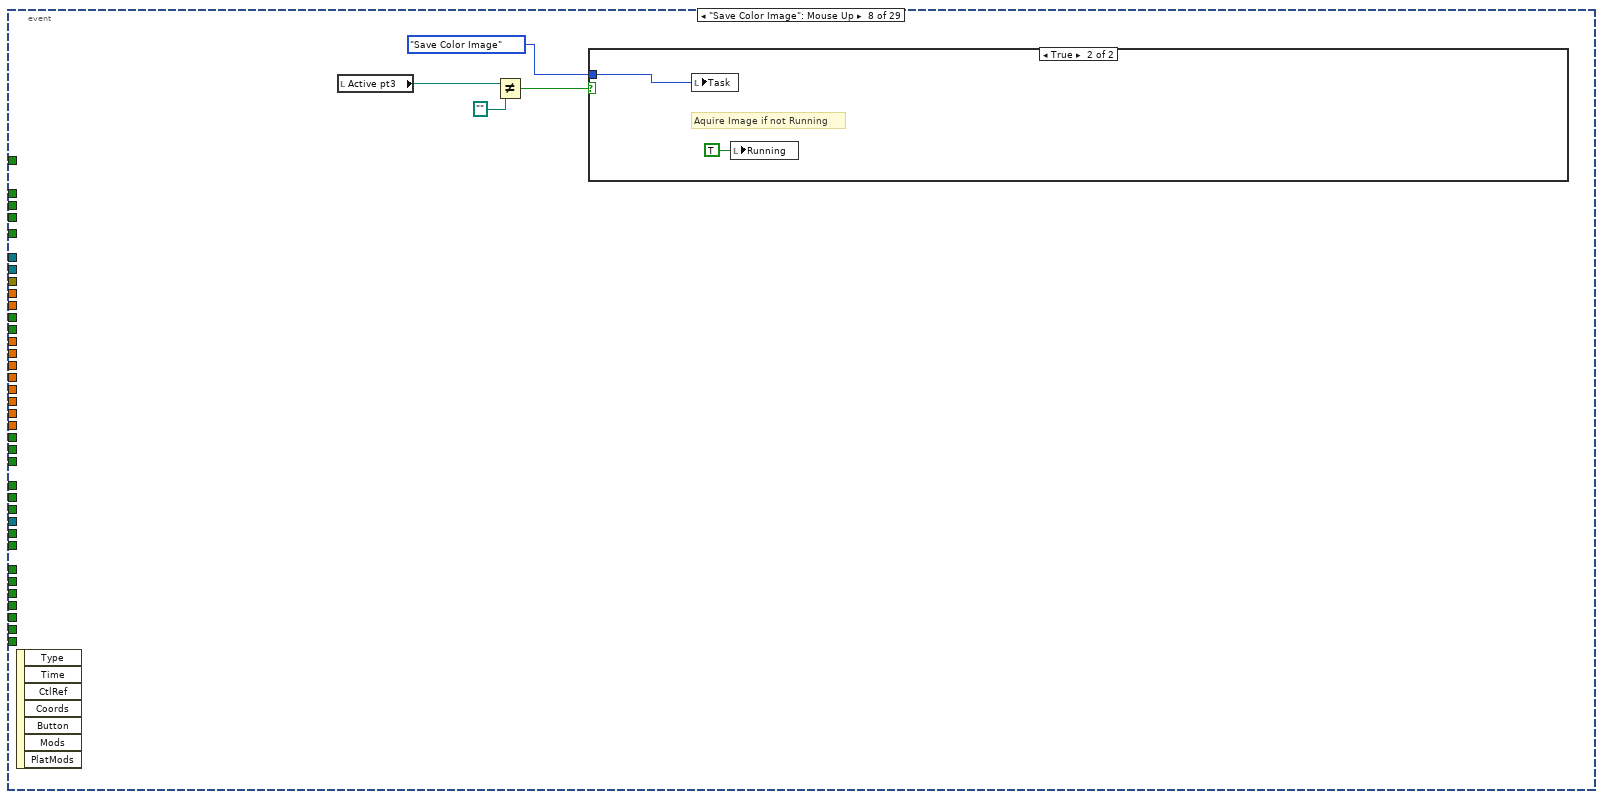
[diagram p19: hidden frame]
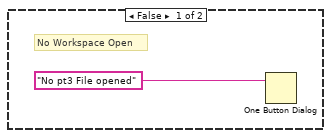
[diagram p20: hidden frame]
diagram:
  n1 = flat-sequence {
    tunnel: [w21] -> w14
    tunnel: errorcluster {"status"=FALSE, "code"=0, "source"=""} ("error in") -> [w32]
    frame #0 {
      (unwired) 1.0 ("CCD Chip Vertical Start")
      w33 = path ""
      w40 = FALSE ("Global Stop")
      n2 = control-ref of="WS File Tree"() -> (w39:refnum<vi>)
      n3 = global write "GetPicture.vi" "GetPicture"(FALSE ("GetPicture")) -> ()
      n4 = local write "Last Image File No"(-1 ("Last Image File No")) -> ()
      n5 = global write "GlobalSetGetConfigureCamera.vi" "gain"(30 ("gain")) -> ()
      n6 = global write "GlobalSetGetConfigureCamera.vi" "Exposure"(sgl 0.1 ("Exposure")) -> ()
      n7 = flat-sequence {
        tunnel: 1.0 ("Vertical Binning") -> [w46]
        tunnel: 1.0 ("CCD Chip Horizontal Start") -> [w45]
        tunnel: 1.0 ("CCD Chip Vertical Start") -> [w41]
        tunnel: 10.0 ("CCD Chip Horizontal End") -> [w44]
        tunnel: 100.0 ("CCD Chip Vertical End") -> [w43]
        tunnel: 1.0 ("Horizontal Binning") -> [w42]
        frame #0 {
          n8 = global write "GlobalSetGetConfigureCamera.vi" "Hbin"(w42) -> ()
          n9 = global write "GlobalSetGetConfigureCamera.vi" "Vbin"(w45) -> ()
          n10 = global write "GlobalSetGetConfigureCamera.vi" "Vbin"(w46) -> ()
          n11 = Subtract(x=w44, y=w45) -> (x-y=w48:dbl)
          n12 = Subtract(x=w43, y=w41) -> (x-y=w47:dbl)
          n13 = global write "ccdChipPixels.vi" "CCD Chip Vertical end"(w43) -> ()
          n14 = global write "ccdChipPixels.vi" "CCD Chip Vertical Start"(w41) -> ()
          n15 = global write "ccdChipPixels.vi" "CCD Chip horizontal end"(w44) -> ()
          n16 = global write "ccdChipPixels.vi" "CCD Chip horizontal start"(w41) -> ()
          n17 = Increment(x=w48) -> (x+1=w50:dbl)
          n18 = Increment(x=w47) -> (x+1=w49:dbl)
          n19 = Multiply(x=w50, y=w49) -> (x*y=w51:dbl)
          n20 = global write "ccdChipPixels.vi" "CCD Chip Size"(w51) -> ()
        }
      }
      n21 = property on="Aquire Image" class="Bool"("BoolText.Text"="Aquire Image" ("Caption.Text"), "BoolText.TextColor"=u32 0 ("Boolean Text.Colors:FG Color")) -> ()  [unwired: 2 in, 2 out]
      n22 = local write "PI SystemNumber"(1 ("PI SystemNumber")) -> ()
      n23 = property on="Point Measurement" class="Bool"("BoolText.Text"="Point Measurement" ("Caption.Text"), "BoolText.TextColor"=u32 0 ("Boolean Text.Colors:FG Color")) -> ()  [unwired: 2 in, 2 out]
      n24 = global write "GlobalCameraHandle.vi" "CameraHandle"(0.0 ("CameraHandle")) -> ()
      n25 = call "MTS_ClearWSTree2.vi"("error in"=w32, "Tree Refnum"=w39) -> ("error out"=w21:errorcluster)  [unwired: 8 in, 1 out]
      "Global Stop" <- w40
      "Running" <- w40
      "Buffer Overrun" <- w40
      "Stop Measurement" <- w40
      "Workspace" <- w33
      "Active pt3" <- w33
      "Task" <- T10."No Measurement" ("Do Measurement")
    }
  }
  n26 = local read "PI SystemNumber"() -> (w9:i32)
  n27 = control-ref of="X-Position"() -> (w13:refnum<vi>)
  n28 = control-ref of="Y-Position"() -> (w12:refnum<vi>)
  n29 = control-ref of="Z-Position"() -> (w11:refnum<vi>)
  n30 = call "AndorPhysikInstrumenteInitialisiation.vi"("reference"=w13, "error in (no error)"=w14, "reference 3"=w11, "reference 2"=w12, "Pi"=w9) -> ("error out"=w6:errorcluster, "Device List"=w18:T12)  [unwired: 5 in]
  n31 = while {
    shift-right: [w55] -> _
    shift-left: w6 -> [w56]
    stop <- w53 stop-if-true
    n32 = Wait (ms)(milliseconds to wait=u32 100) -> ()  [unwired: 1 out]
    n33 = local read "Global Stop"() -> (w53:bool)
    n34 = control-ref of="Point"() -> (w52:refnum<vi>)
    n35 = call "RunCameraPreview.vi"("error in (no error)"=w56, "Point 2"=w52) -> ("error out"=w55:errorcluster)  [unwired: 9 in]
  }
  n36 = while {
    tunnel: w6 -> [w73]
    stop <- w59 stop-if-true
    n37 = local read "Global Stop"() -> (w74:bool)
    n38 = local read "Global Stop"() -> (w59:bool)
    n39 = call "Vision Acquisition"("Auto Exposure::Mode"="Auto Exposure::Mode", "Auto Exposure::Value"="Auto Exposure::Value", "Brightness::Mode"="Brightness::Mode", "Brightness::Value"="Brightness::Value", "Gain::Mode"="Gain::Mode", "Stop (F)"=w74, "Gain::Value"="Gain::Value", "error in"=w73, "Gamma::Mode"="Gamma::Mode", "Shutter::Mode"="Shutter::Mode", "Shutter::Value"="Shutter::Value", "Trigger::Trigger Activation"="Trigger::Trigger Activation", "Trigger::Trigger Mode"="Trigger::Trigger Mode", "Trigger::Trigger Parameter"="Trigger::Trigger Parameter", "Trigger Delay::Mode"="Trigger Delay::Mode") -> ("Image Out"=→"Image Out":T5, "Image Number"=→"Image Number":u32, "Frame Rate"=→"acquired FPS":dbl)  [unwired: 8 in, 2 out]
  }
  n40 = while {
    shift-right: [w114] -> _
    shift-left: w6 -> [w116]
    stop <- w115 stop-if-true
    n41 = local read "Global Stop"() -> (w115:bool)
    n42 = control-ref of="WS File Tree"() -> (w89:refnum<vi>)
    n43 = global read "GlobalLaserInterface.vi" "InterfaceLaserInitalised"() -> (w77:refnum<visa-resource-name>)
    n44 = event shown="[19] \"Set Temperature\": Value Change" {
      selector: _ -> [_ _ _ _ _ _ _ _ _ _ _ _ _ _ _ _ _ _ _ _ _ _ _ _ _ _ _ _ _]
      dyn-events: _ -> [_ _ _ _ _ _ _ _ _ _ _ _ _ _ _ _ _ _ _ _ _ _ _ _ _ _ _ _ _]
      timeout: _ -> [_ _ _ _ _ _ _ _ _ _ _ _ _ _ _ _ _ _ _ _ _ _ _ _ _ _ _ _ _]
      tunnel: w116 -> [w117 w119 _ _ w194 _ w237 _ _ _ w280 w333 w336 w372 _ w432 _ w472 w479 w508 _ w518 w527 w538 w540 _ _ _ w547]
      tunnel: [w117 w119 _ _ w195 _ w236 _ _ _ w279 w325 w334 w369 _ w431 _ w471 _ _ _ w516 _ w537 _ _ _ _ w548] -> w114
      tunnel: w89 -> [_ _ _ _ _ _ _ _ _ _ _ _ w338 w373 _ _ _ _ _ _ _ _ _ _ _ _ _ _ _]
      tunnel: "Aquire Image" -> [_ _ _ _ _ _ _ _ _ _ _ _ _ _ _ _ _ _ _ _ _ _ _ _ _ _ _ _ _]
      tunnel: "Save Color Image" -> [_ _ _ _ _ _ _ _ _ _ _ _ _ _ _ _ _ _ _ _ _ _ _ _ _ _ _ _ _]
      tunnel: "Open MSW" -> [_ _ _ _ _ _ _ _ _ _ _ _ _ _ _ _ _ _ _ _ _ _ _ _ _ _ _ _ _]
      tunnel: "Find Mols" -> [_ _ _ _ _ _ _ _ _ _ _ _ _ _ _ _ _ _ _ _ _ _ _ _ _ _ _ _ _]
      tunnel: "Auto Meas" -> [_ _ _ _ _ _ _ _ _ _ _ _ _ _ _ _ _ _ _ _ _ _ _ _ _ _ _ _ _]
      tunnel: "New MSW" -> [_ _ _ _ _ _ _ _ _ _ _ _ _ _ _ _ _ _ _ _ _ _ _ _ _ _ _ _ _]
      tunnel: "Stop Program" -> [_ _ _ _ _ _ _ _ _ _ _ _ _ _ _ _ _ _ _ _ _ _ _ _ _ _ _ _ _]
      tunnel: "Point Measurement" -> [_ _ _ _ _ _ _ _ _ _ _ _ _ _ _ _ _ _ _ _ _ _ _ _ _ _ _ _ _]
      tunnel: "Move Stage" -> [_ _ _ _ _ _ _ _ _ _ _ _ _ _ _ _ _ _ _ _ _ _ _ _ _ _ _ _ _]
      tunnel: w77 -> [_ _ _ _ _ _ _ _ _ _ _ _ _ _ _ _ _ _ _ _ _ _ _ _ _ _ _ _ _]
      tunnel: "Get Position" -> [_ _ _ _ _ _ _ _ _ _ _ _ _ _ _ _ _ _ _ _ _ _ _ _ _ _ _ _ _]
      tunnel: [_ _ _ _ _ _ _ _ _ _ w275 w318 _ _ _ _ _ _ _ _ _ _ _ _ _ _ _ _ _] -> w104
      tunnel: [_ _ _ _ _ _ _ _ _ _ w276 w319 _ _ _ _ _ _ _ _ _ _ _ _ _ _ _ _ _] -> w88
      tunnel: [_ _ _ _ _ _ _ _ _ _ w277 w320 _ _ _ _ _ _ _ _ _ _ _ _ _ _ _ _ _] -> w103
      tunnel: "How long?" -> [_ _ _ _ _ _ _ _ _ _ _ _ _ _ _ _ _ _ _ _ _ _ _ _ _ _ _ _ _]
      tunnel: "Start 3D FCS Abel Scan" -> [_ _ _ _ _ _ _ _ _ _ _ _ _ _ _ _ _ _ _ _ _ _ _ _ _ _ _ _ _]
      tunnel: "Mesaurement Time (Sec) / Step" -> [_ _ _ w153 w199 _ _ _ _ _ _ _ _ _ _ _ _ _ _ _ _ _ _ _ _ _ w545 _ _]
      tunnel: "Y Stepsize" -> [_ _ _ w152 w198 _ _ _ _ _ _ _ _ _ _ _ _ _ _ _ _ _ _ _ _ _ _ _ _]
      tunnel: "X Stepsize" -> [_ _ _ w151 w197 _ _ _ _ _ _ _ _ _ _ _ _ _ _ _ _ _ _ _ _ _ _ _ _]
      tunnel: "Z Stepsize" -> [_ _ _ w150 w196 _ _ _ _ _ _ _ _ _ _ _ _ _ _ _ _ _ _ _ _ _ _ _ _]
      tunnel: "FCS Point Measurement" -> [_ _ _ _ _ _ _ _ _ _ _ _ _ _ _ _ _ _ _ _ _ _ _ _ _ _ _ _ _]
      tunnel: "Z End" -> [_ _ _ w149 w208 _ _ _ _ _ _ _ _ _ _ _ _ _ _ _ _ _ _ _ _ _ _ _ _]
      tunnel: "X End" -> [_ _ _ w148 w202 _ _ _ _ _ _ _ _ _ _ _ _ _ _ _ _ _ _ _ _ _ _ _ _]
      tunnel: "Y End" -> [_ _ _ w147 w205 _ _ _ _ _ _ _ _ _ _ _ _ _ _ _ _ _ _ _ _ _ _ _ _]
      tunnel: "Z Start" -> [_ _ _ w146 w188 _ _ _ _ _ _ _ _ _ _ _ _ _ _ _ _ _ _ _ _ _ _ _ _]
      tunnel: "X Start" -> [_ _ _ w145 w190 _ _ _ _ _ _ _ _ _ _ _ _ _ _ _ _ _ _ _ _ _ _ _ _]
      tunnel: "Y Start" -> [_ _ _ w144 w189 _ _ _ _ _ _ _ _ _ _ _ _ _ _ _ _ _ _ _ _ _ _ _ _]
      tunnel: w89 -> [_ _ _ _ _ _ _ _ _ _ _ _ _ _ _ _ _ _ _ _ _ _ _ _ _ _ _ _ _]
      tunnel: "SET CCD" -> [_ _ _ _ _ _ _ _ _ _ _ _ _ _ _ _ _ _ _ _ _ _ _ _ _ _ _ _ _]
      tunnel: "OPEN SHUTER" -> [_ _ _ _ _ _ _ _ _ _ _ _ _ _ _ _ _ _ _ _ _ w517 _ _ _ _ _ _ _]
      tunnel: "Close" -> [_ _ _ _ _ _ _ _ _ _ _ _ _ _ _ _ _ _ _ _ _ _ w526 _ _ _ _ _ _]
      tunnel: "Stop" -> [_ _ _ _ _ _ _ _ _ _ _ _ _ _ _ _ _ _ _ _ _ _ _ _ _ _ _ _ _]
      tunnel: "Start" -> [_ _ _ _ _ _ _ _ _ _ _ _ _ _ _ _ _ _ _ _ _ _ _ _ _ _ _ _ _]
      tunnel: "Gain" -> [_ _ _ _ _ _ _ _ _ _ _ _ _ _ _ _ _ _ _ _ _ _ _ _ _ _ _ _ _]
      tunnel: "Cam (Defocused)" -> [_ _ _ _ _ _ _ _ _ _ _ _ _ _ _ _ _ _ _ _ w515 _ _ _ _ _ _ _ _]
      tunnel: "Set Temperature" -> [_ _ _ _ _ _ _ _ _ _ _ _ _ _ _ _ _ _ _ _ _ _ _ _ _ _ _ _ _]
      tunnel: "SCANNER EMERGENCY" -> [_ _ _ _ _ _ _ _ _ _ _ _ _ _ _ _ _ _ _ _ _ _ _ _ _ _ _ _ _]
      tunnel: "Get Temperature" -> [_ _ _ _ _ _ _ _ _ _ _ _ _ _ _ _ _ _ _ _ _ _ _ _ _ _ _ _ _]
      event Timeout {
        n45 = event-data() -> ()  [unwired: 1 in, 2 out]
      }
      event "Stop Program": Mouse Up {
        n46 = event-data() -> ()  [unwired: 1 in, 7 out]
        n47 = local write "Global Stop"(TRUE ("Global Stop")) -> ()
      }
      event "Aquire Image": Mouse Up {
        n48 = event-data() -> ()  [unwired: 1 in, 7 out]
        n49 = local read "Workspace"() -> (w123:path)
        n50 = local read "Running"() -> (w126:bool)
        n51 = Not(x=w126) -> (.not. x?=w125:bool)
        n52 = Not Equal?(x=w123, y=path "") -> (x != y?=w121:bool)
        n53 = local read "Task"() -> (w120:T10)
        n54 = case shown="True" w121 {
          tunnel: w125 -> [_ w130]
          tunnel: T13."Aquire Image" ("Do Measurement") -> [_ w129]
          tunnel: w120 -> [_ w128]
          frame False {
            # "No Workspace Open"
            n55 = One Button Dialog(message="No Workspace Opened") -> ()  [unwired: 1 in, 1 out]
          }
          frame True {
            # "Aquire Image if not Running"
            n56 = case shown="True" w130 {
              tunnel: w129 -> [w133 w136]
              tunnel: w128 -> [w131 _]
              frame False {
                n57 = Equal?(x=w131, y=w133) -> (x = y?=w132:bool)
                n58 = case shown="False" w132 {
                  frame False {
                  }
                  frame True {
                    n59 = local write "Stop Measurement"(TRUE ("Stop Measurement")) -> ()
                  }
                }
              }
              frame True {
                n60 = local write "Task"(w136) -> ()
                n61 = local write "Running"(TRUE ("Measurement Running")) -> ()
                n62 = property on="Aquire Image" class="Bool"("BoolText.Text"="Stop Aquire" ("Caption.Text"), "BoolText.TextColor"=u32 16711680 ("Boolean Text.Colors:FG Color")) -> ()  [unwired: 2 in, 2 out]
              }
            }
          }
        }
      }
      event "How long?": Value Change {
        n63 = event-data() -> ()  [unwired: 1 in, 5 out]
        n64 = Build Array(w153, w152, w151, w150, w149, w148, w147, w146, w145, w144) -> (w143:dbl[])
        n65 = for {
          tunnel: w143 -> [w181] mode=indexing
          tunnel: [w180] -> w142 mode=indexing
          n66 = Not Equal To 0?(x=w181) -> (x != 0?=w180:bool)
        }
        n67 = Boolean Array To Number(Boolean array=w142) -> (number=w141:u32)
        n68 = Not Equal To 0?(x=w141) -> (x != 0?=w140:bool)
        n69 = case shown="True" w140 {
          tunnel: [0.0 w166] -> w139
          tunnel: w153 -> [_ w165]
          tunnel: w152 -> [_ w164]
          tunnel: w151 -> [_ w163]
          tunnel: w150 -> [_ w162]
          tunnel: w149 -> [_ w161]
          tunnel: w148 -> [_ w160]
          tunnel: w147 -> [_ w159]
          tunnel: w146 -> [_ w158]
          tunnel: w145 -> [_ w157]
          tunnel: w144 -> [_ w156]
          frame False {
            n70 = One Button Dialog(message="Supply valid information for the scanner x-z and stepsize and apply a measurement time ") -> ()  [unwired: 1 in, 1 out]
          }
          frame True {
            w167 = 60.0 ("y")
            # "to hours"
            # "to minutes"
            n71 = Subtract(x=w161, y=w158) -> (x-y=w174:dbl)
            n72 = Subtract(x=w160, y=w157) -> (x-y=w179:dbl)
            n73 = Subtract(x=w159, y=w156) -> (x-y=w176:dbl)
            n74 = Divide(x=w174, y=w162) -> (x/y=w175:dbl)
            n75 = Divide(x=w179, y=w163) -> (x/y=w178:dbl)
            n76 = Divide(x=w176, y=w164) -> (x/y=w177:dbl)
            n77 = Multiply(x=w165, y=w175) -> (x*y=w171:dbl)
            n78 = Multiply(x=w165, y=w178) -> (x*y=w173:dbl)
            n79 = Multiply(x=w165, y=w177) -> (x*y=w172:dbl)
            n80 = Add(x=w173, y=w172) -> (x+y=w170:dbl)
            n81 = Add(x=w171, y=w170) -> (x+y=w169:dbl)
            n82 = Divide(x=w169, y=w167) -> (x/y=w168:dbl)
            n83 = Divide(x=w168, y=w167) -> (x/y=w166:dbl)
          }
        }
        "Estimated Time (h)" <- w139
      }
      event "Start 3D FCS Abel Scan": Value Change {
        w191 = 200
        n84 = event-data() -> ()  [unwired: 1 in, 5 out]
        n85 = local write "Z Stepsize"(w196) -> ()
        n86 = local write "X-Position"(w190) -> ()
        n87 = local write "Y-Position"(w189) -> ()
        n88 = local write "Y Stepsize"(w198) -> ()
        n89 = property on="Measurement Time" class="DigNum (strict)"("Value"=w199) -> ()  [unwired: 2 in, 2 out]
        n90 = local write "Z-Position"(w188) -> ()
        n91 = local write "X Stepsize"(w197) -> ()
        n92 = case shown="No Error" w194 {
          selector: w194 -> [w209 w211]
          tunnel: [w209 w211] -> w183
          frame No Error {
            n93 = global write "StopGetPic.vi" "Stop"(TRUE ("Stop")) -> ()
          }
          frame Error {
          }
        }
        n94 = Subtract(x=w202, y=w190) -> (x-y=w201:dbl)
        n95 = Subtract(x=w208, y=w188) -> (x-y=w206:dbl)
        n96 = Subtract(x=w205, y=w189) -> (x-y=w204:dbl)
        n97 = Divide(x=w201, y=w197) -> (x/y=→"X Steps":dbl)
        n98 = Divide(x=w206, y=w196) -> (x/y=→"Z Steps":dbl)
        n99 = Divide(x=w204, y=w198) -> (x/y=→"Y Steps":dbl)
        n100 = local read "PI SystemNumber"() -> (w193:i32)
        n101 = Subtract(x=w191, y=w188) -> (x-y=w185:dbl)
        n102 = Subtract(x=w191, y=w189) -> (x-y=w186:dbl)
        n103 = Subtract(x=w191, y=w190) -> (x-y=w187:dbl)
        n104 = Build Array(w187, w186, w185) -> (w184:dbl[])
        n105 = global read "GlobalConAxisPI.vi" "Conn. Axes"() -> (w192:string[])
        n106 = call "MOV.vi"("System no."=w193, "Axes to move"=w192, "Position values"=w184, "error in"=w183) -> ("error out"=w182:errorcluster)  [unwired: 15 in]
        n107 = case shown="No Error" w182 {
          selector: w182 -> [w212 w214]
          tunnel: [w212 w214] -> w195
          frame No Error {
            "3dAbelFcs" <- TRUE
          }
          frame Error {
          }
        }
      }
      event "Auto Meas": Mouse Up {
        n108 = event-data() -> ()  [unwired: 1 in, 7 out]
        n109 = local read "Workspace"() -> (w222:path)
        n110 = local read "Running"() -> (w225:bool)
        n111 = local read "Last Image File No"() -> (w219:i32)
        n112 = Not(x=w225) -> (.not. x?=w224:bool)
        n113 = Not Equal?(x=w222, y=path "") -> (x != y?=w217:bool)
        n114 = Not Equal?(x=w219, y=-1) -> (x != y?=w216:bool)
        n115 = And(x=w217, y=w216) -> (x .and. y?=w215:bool)
        n116 = local read "Task"() -> (w223:T10)
        n117 = case shown="False" w215 {
          tunnel: w224 -> [_ w229]
          tunnel: T14."Auto Measurement Control" ("Do Measurement") -> [_ w228]
          tunnel: w223 -> [_ w227]
          frame False {
            # "No Workspace Open"
            n118 = One Button Dialog(message="No Workspace Opened or No Image Acquired") -> ()  [unwired: 1 in, 1 out]
          }
          frame True {
            # "Start Auto Measurement"
            n119 = case shown="True" w229 {
              tunnel: w228 -> [_ w233]
              tunnel: w227 -> [_ _]
              frame False {
                n120 = case shown="True" FALSE {
                  frame False {
                  }
                  frame True {
                    n121 = local write "Stop Measurement"(TRUE ("Stop Measurement")) -> ()
                  }
                }
              }
              frame True {
                n122 = local write "Task"(w233) -> ()
                n123 = local write "Running"(TRUE ("Measurement Running")) -> ()
                n124 = local write "NxtAutMesPoint"(-1 ("NxtAutMesPoint")) -> ()
              }
            }
          }
        }
      }
      event "Get Temperature": Value Change {
        n125 = event-data() -> ()  [unwired: 1 in, 5 out]
        n126 = call "GetTemperature.vi"("error in (no error)"=w237) -> ("error out"=w238:errorcluster, "temperature"=w241:i32)  [unwired: 3 in, 2 out]
        n127 = call "Build Text"("Cam"=w241, "error in (no error)"=w238) -> ("Result"=w240:string, "error out"=w239:errorcluster)  [unwired: 12 in]
        n128 = call "Display Message to User"("error in (no error)"=w239, "Enable"=TRUE, "Message"=w240) -> ("error out"=w236:errorcluster)  [unwired: 7 in, 1 out]
      }
      event "Save Color Image": Mouse Up {
        n129 = event-data() -> ()  [unwired: 1 in, 7 out]
        n130 = local read "Active pt3"() -> (w244:path)
        n131 = Not Equal?(x=w244, y=path "") -> (x != y?=w242:bool)
        n132 = case shown="True" w242 {
          tunnel: T15."Save Color Image" ("Do Measurement") -> [_ w248]
          frame False {
            # "No Workspace Open"
            n133 = One Button Dialog(message="No pt3 File opened") -> ()  [unwired: 1 in, 1 out]
          }
          frame True {
            # "Aquire Image if not Running"
            n134 = local write "Task"(w248) -> ()
            n135 = local write "Running"(TRUE ("Measurement Running")) -> ()
          }
        }
      }
      event "Find Mols": Mouse Up {
        n136 = event-data() -> ()  [unwired: 1 in, 7 out]
        n137 = local read "Active pt3"() -> (w251:path)
        n138 = Not Equal?(x=w251, y=path "") -> (x != y?=w249:bool)
        n139 = case shown="True" w249 {
          tunnel: T15."Find Single Mol." ("Do Measurement") -> [_ w255]
          frame False {
            # "No Workspace Open"
            n140 = One Button Dialog(message="No pt3 File opened") -> ()  [unwired: 1 in, 1 out]
          }
          frame True {
            # "Aquire Image if not Running"
            n141 = local write "Task"(w255) -> ()
            n142 = local write "Running"(TRUE ("Measurement Running")) -> ()
          }
        }
      }
      event "Point Measurement": Mouse Up {
        n143 = event-data() -> ()  [unwired: 1 in, 7 out]
        n144 = local read "Workspace"() -> (w258:path)
        n145 = local read "Running"() -> (w262:bool)
        n146 = Not(x=w262) -> (.not. x?=w261:bool)
        n147 = Not Equal?(x=w258, y=path "") -> (x != y?=w256:bool)
        n148 = local read "Task"() -> (w259:T10)
        n149 = case shown="True" w256 {
          tunnel: w261 -> [_ w266]
          tunnel: T13."Point Measurement" ("Do Measurement") -> [_ w265]
          tunnel: w259 -> [_ w264]
          frame False {
            # "No Workspace Open"
            n150 = One Button Dialog(message="No Workspace Opened") -> ()  [unwired: 1 in, 1 out]
          }
          frame True {
            # "Aquire Image if not Running"
            n151 = case shown="False" w266 {
              tunnel: w265 -> [w268 w272]
              tunnel: w264 -> [w269 _]
              frame False {
                n152 = Equal?(x=w269, y=w268) -> (x = y?=w267:bool)
                n153 = case shown="False" w267 {
                  frame False {
                  }
                  frame True {
                    n154 = local write "Stop Measurement"(TRUE ("Stop Measurement")) -> ()
                  }
                }
              }
              frame True {
                n155 = local write "Task"(w272) -> ()
                n156 = local write "Running"(TRUE ("Measurement Running")) -> ()
                n157 = property on="Point Measurement" class="Bool"("BoolText.Text"="Stop Aquire" ("Caption.Text"), "BoolText.TextColor"=u32 16711680 ("Boolean Text.Colors:FG Color")) -> ()  [unwired: 2 in, 2 out]
              }
            }
          }
        }
      }
      event "X-Position", "Y-Position", "Z-Position": Value Change; "Move Stage": Mouse Up {
        n158 = event-data() -> ()  [unwired: 1 in, 3 out]
        n159 = local read "Workspace"() -> (w283:path)
        n160 = local read "Running"() -> (w285:bool)
        n161 = local read "PI SystemNumber"() -> (w278:i32)
        n162 = Not(x=w285) -> (.not. x?=w284:bool)
        n163 = Not Equal?(x=w283, y=path "") -> (x != y?=w281:bool)
        n164 = case shown="True" w281 {
          tunnel: w284 -> [_ w293]
          tunnel: w280 -> [_ w292]
          tunnel: [_ w291] -> w279
          tunnel: w278 -> [_ w290]
          tunnel: [_ w289] -> w275
          tunnel: [_ w288] -> w276
          tunnel: [_ w287] -> w277
          frame False {
            # "No Workspace Open"
            n165 = One Button Dialog(message="No Workspace Opened") -> ()  [unwired: 1 in, 1 out]
          }
          frame True {
            # "Move Stage if not Running"
            n166 = case shown="True" w293 {
              tunnel: w292 -> [_ w317]
              tunnel: [_ w307] -> w291
              tunnel: w290 -> [_ w315]
              tunnel: [_ w294] -> w289
              tunnel: [_ w295] -> w288
              tunnel: [_ w296] -> w287
              frame False {
              }
              frame True {
                w299 = 200
                n167 = local read "X-Position"() -> (w302:dbl)
                n168 = local read "Y-Position"() -> (w301:dbl)
                n169 = local read "Z-Position"() -> (w306:dbl)
                n170 = Subtract(x=w299, y=w302) -> (x-y=w303:dbl)
                n171 = Subtract(x=w299, y=w301) -> (x-y=w304:dbl)
                n172 = Subtract(x=w299, y=w306) -> (x-y=w305:dbl)
                n173 = Build Array(w303, w304, w305) -> (w316:dbl[])
                n174 = global read "GlobalConAxisPI.vi" "Conn. Axes"() -> (w314:string[])
                n175 = call "MOV.vi"("System no."=w315, "Axes to move"=w314, "Position values"=w316, "error in"=w317) -> ("error out"=w312:errorcluster)  [unwired: 15 in]
                n176 = call "POS?.vi"("System no."=w315, "Axes to query"=w314, "All axes?"=TRUE, "error in"=w312) -> ("Position"=w311:dbl[], "error out"=w307:errorcluster)  [unwired: 14 in]
                n177 = Index Array(array=w311, index #1=0 ("index"), index #2=1 ("index"), index #3=2 ("index")) -> (element #1=w300:dbl, element #2=w297:dbl, element #3=w298:dbl)
                n178 = Subtract(x=w299, y=w300) -> (x-y=w296:dbl)
                n179 = Subtract(x=w299, y=w297) -> (x-y=w295:dbl)
                n180 = Subtract(x=w299, y=w298) -> (x-y=w294:dbl)
              }
            }
          }
        }
        n181 = property on="y-position" class="DigNum (strict)"("Value"=w276) -> ()  [unwired: 2 in, 2 out]
        n182 = property on="z-position" class="DigNum (strict)"("Value"=w275) -> ()  [unwired: 2 in, 2 out]
        n183 = property on="x-position" class="DigNum (strict)"("Value"=w277) -> ()  [unwired: 2 in, 2 out]
      }
      event "Get Position": Value Change {
        w324 = 200
        n184 = event-data() -> ()  [unwired: 1 in, 5 out]
        n185 = local read "PI SystemNumber"() -> (w332:i32)
        n186 = global read "GlobalConAxisPI.vi" "Conn. Axes"() -> (w331:string[])
        n187 = call "POS?.vi"("System no."=w332, "Axes to query"=w331, "All axes?"=TRUE, "error in"=w333) -> ("Position"=w329:dbl[], "error out"=w325:errorcluster)  [unwired: 14 in]
        n188 = Index Array(array=w329, index #1=0 ("index"), index #2=1 ("index"), index #3=2 ("index")) -> (element #1=w321:dbl, element #2=w322:dbl, element #3=w323:dbl)
        n189 = Subtract(x=w324, y=w321) -> (x-y=w320:dbl)
        n190 = Subtract(x=w324, y=w322) -> (x-y=w319:dbl)
        n191 = Subtract(x=w324, y=w323) -> (x-y=w318:dbl)
        n192 = property on="y-position" class="DigNum (strict)"("Value"=w319) -> ()  [unwired: 2 in, 2 out]
        n193 = property on="x-position" class="DigNum (strict)"("Value"=w320) -> ()  [unwired: 2 in, 2 out]
        n194 = property on="z-position" class="DigNum (strict)"("Value"=w318) -> ()  [unwired: 2 in, 2 out]
      }
      event "New MSW": Mouse Up {
        # "Default Name"
        n195 = event-data() -> ()  [unwired: 1 in, 7 out]
        n196 = flat-sequence {
          tunnel: [w354] -> w337
          tunnel: w336 -> [w354]
          frame #0 {
            n197 = local write "Running"(TRUE ("MeasRunig")) -> ()
          }
        }
        n198 = Get Date/Time In Seconds() -> (seconds since 1Jan1904=w351:timestamp)
        n199 = Format Date/Time String(time format string (%c)="%Y-%m-%d", seconds (now)=w351) -> (date/time string=w349:string)  [unwired: 1 out]
        n200 = Concatenate Strings(w349, ".msw" ("string")) -> (w347:string)
        n201 = call "File Dialog"("start path"=path "D:/", "prompt"="Create New Workspace", "button label"="Create", "default name"=w347, "error in"=w337, "pattern (all files)"="*.msw", "pattern label"="MT Scan Workspace") -> ("selected path"=w341:path, "cancelled"=w342:bool, "error out"=w340:errorcluster)  [unwired: 5 in, 1 out]
        n202 = case shown="False" w342 {
          tunnel: w341 -> [w360 _]
          tunnel: w340 -> [w366 w368]
          tunnel: [w358 w367] -> w335
          tunnel: w338 -> [w356 _]
          frame False {
            # "Create Empty Workspace"
            n203 = local write "Workspace"(w360) -> ()
            n204 = call "MTS_CreateWriteMSW.vi"("Rewrite"=TRUE, "error in (no error)"=w366, "Workspace Path"=w360) -> ("error out"=w359:errorcluster, "Created"=w363:string, "Comment (dup)"=w362:string, "Files in Workspace (dup)"=w361:T19)  [unwired: 5 in]
            n205 = call "MTS_Workspace.vi"("Workspace"=w360, "Operation"=T16."Set Workspace", "Created in"=w363, "New Comment"=w362, "Files in Workspace in"=w361) -> ("Files in Workspace"=w357:T20)  [unwired: 3 in, 3 out]
            n206 = call "MTS_BuildWSTree.vi"("error in"=w359, "Files in Workspace"=w357, "Tree Refnum"=w356) -> ("error out"=w358:errorcluster)  [unwired: 6 in, 2 out]
          }
          frame True {
            n207 = call <vilib>:"Clear Errors.vi"("error in (no error)"=w368) -> ("error out"=w367:errorcluster)  [unwired: 6 in]
          }
        }
        n208 = flat-sequence {
          tunnel: w335 -> [w352]
          tunnel: [w352] -> w334
          frame #0 {
            n209 = local write "Running"(FALSE ("MeasRunig")) -> ()
          }
        }
      }
      event "Open MSW": Mouse Up {
        n210 = event-data() -> ()  [unwired: 1 in, 7 out]
        n211 = flat-sequence {
          tunnel: w372 -> [w384]
          tunnel: [w384] -> w371
          frame #0 {
            n212 = local write "Running"(TRUE ("MeasRunig")) -> ()
          }
        }
        n213 = call "File Dialog2"("start path"=path "D:/", "prompt"="Create New Workspace", "button label"="Open", "error in"=w371, "pattern (all files)"="*.msw", "pattern label"="MT Scan Workspace") -> ("selected path"=w376:path, "cancelled"=w377:bool, "error out"=w375:errorcluster)  [unwired: 6 in, 1 out]
        n214 = case shown="False" w377 {
          tunnel: w376 -> [w392 _]
          tunnel: w375 -> [w397 w399]
          tunnel: [w390 w398] -> w370
          tunnel: w373 -> [w389 _]
          frame False {
            # "Open Workspace"
            n215 = local write "Workspace"(w392) -> ()
            n216 = call "MTS_ReadMSW.vi"("error in (no error)"=w397, "Workspace Path"=w392) -> ("error out"=w391:errorcluster, "Created"=w395:string, "Comment"=w394:string, "Files in Workspace"=w393:T21)  [unwired: 6 in]
            n217 = call "MTS_Workspace.vi"("Workspace"=w392, "Operation"=T16."Set Workspace", "Created in"=w395, "New Comment"=w394, "Files in Workspace in"=w393) -> ("Files in Workspace"=w388:T20)  [unwired: 3 in, 3 out]
            n218 = Array To Cluster(array=w388) -> (cluster=w387:T22)
            n219 = Unbundle By Name(w387) -> ()  [unwired: 1 out]
            n220 = call "MTS_BuildWSTree.vi"("error in"=w391, "Files in Workspace"=w388, "Tree Refnum"=w389) -> ("error out"=w390:errorcluster, "numberOfFilesInWorkspace"=w386:i32)  [unwired: 6 in, 1 out]
            n221 = local write "Last Image File No"(w386) -> ()
          }
          frame True {
            n222 = call <vilib>:"Clear Errors.vi"("error in (no error)"=w399) -> ("error out"=w398:errorcluster)  [unwired: 6 in]
          }
        }
        n223 = flat-sequence {
          tunnel: w370 -> [w382]
          tunnel: [w382] -> w369
          frame #0 {
            n224 = local write "Running"(FALSE ("MeasRunig")) -> ()
          }
        }
      }
      event "Image": Mouse Up {
        w402 = 100.0 ("y")
        n225 = event-data() -> ("Coords"=w414:T23, "PlatMods"=w415:T24)  [unwired: 1 in, 5 out]
        n226 = invoke on="Image" class="IntGraph (strict)" method="Map Coords To XY"("Coords"=w414) -> ("Map Coords To XY"=w411:bool, "XY"=w409:cluster{"X":dbl, "Y":dbl})  [unwired: 6 in, 5 out]
        n227 = Unbundle By Name(w415) -> ("Ctrl"=w412:bool)
        n228 = And(x=w411, y=w412) -> (x .and. y?=w413:bool)
        n229 = Unbundle(w409) -> ("X"=w408:dbl, "Y"=w405:dbl)
        n230 = Multiply(x=w408, y=w402) -> (x*y=w407:dbl)
        n231 = Multiply(x=w405, y=w402) -> (x*y=w404:dbl)
        n232 = Round To Nearest(number=w407) -> (nearest integer value=w406:dbl)
        n233 = Round To Nearest(number=w404) -> (nearest integer value=w403:dbl)
        n234 = Divide(x=w406, y=w402) -> (x/y=w401:dbl)
        n235 = Divide(x=w403, y=w402) -> (x/y=w400:dbl)
        n236 = local read "Axis"() -> (w410:enum32{"x-y", "x-z", "y-x", "y-z", "z-x", "z-y"})
        n237 = case shown="True" w413 {
          tunnel: w410 -> [_ w418]
          tunnel: w401 -> [_ w417]
          tunnel: w400 -> [_ w416]
          frame False {
          }
          frame True {
            n238 = case shown="\"x-y\", Default" w418 {
              tunnel: w417 -> [w420 w422 w424]
              tunnel: w416 -> [w419 w421 w423]
              frame "x-y", Default {
                n239 = local write "X-Position"(w420) -> ()
                n240 = local write "Y-Position"(w419) -> ()
              }
              frame "x-z" {
                n241 = local write "X-Position"(w422) -> ()
                n242 = local write "Z-Position"(w421) -> ()
              }
              frame "y-z" {
                n243 = local write "Y-Position"(w424) -> ()
                n244 = local write "Z-Position"(w423) -> ()
              }
            }
          }
        }
      }
      event "WS File Tree": Value Change {
        n245 = event-data() -> ("NewVal"=w433:string)  [unwired: 1 in, 4 out]
        n246 = control-ref of="Workspace"() -> (w430:refnum<vi>)
        n247 = control-ref of="Histogram"() -> (w428:refnum<vi>)
        n248 = control-ref of="Trace"() -> (w427:refnum<vi>)
        n249 = control-ref of="Image"() -> (w426:refnum<vi>)
        n250 = control-ref of="Image"() -> (w425:refnum<vi>)
        n251 = control-ref of="Active pt3"() -> (w429:refnum<vi>)
        n252 = call "CreateNewWSfile.vi"("reference 5"=w425, "NewVal"=w433, "Image"=w426, "reference in"=w429, "error in (no error)"=w432, "reference 4"=w427, "reference 3"=w428, "Path in"=w430) -> ("error out"=w431:errorcluster)  [unwired: 3 in]
      }
      event "Resolution", "Picture size", "Pixel time", "Picture size 2", "Axis", "Laser  Profile": Value Change {
        n253 = event-data() -> ()  [unwired: 1 in, 5 out]
        n254 = local read "Axis"() -> (w454:enum32{"x-y", "x-z", "y-x", "y-z", "z-x", "z-y"})
        n255 = local read "Picture size"() -> (w456:dbl)
        n256 = local read "X-Position"() -> (w451:dbl)
        n257 = local read "Y-Position"() -> (w450:dbl)
        n258 = local read "Z-Position"() -> (w449:dbl)
        n259 = local read "Resolution"() -> (w448:dbl)
        n260 = local read "Pixel time"() -> (w457:dbl)
        n261 = local write "Axis"(w454) -> ()
        n262 = local read "Picture size 2"() -> (w455:dbl)
        n263 = local read "Laser  Profile"() -> (w438:string)
        n264 = local write "Pixel time"(w457) -> ()
        n265 = call "PI_CheckScan.vi"("Picture size"=w456, "Picture size 2"=w455, "Axis"=w454, "x-Position"=w451, "y-Position"=w450, "z-Position"=w449) -> ("Picture size out"=w452:dbl, "Picture size out 2"=w453:dbl)  [unwired: 8 in, 4 out]
        n266 = String To Byte Array(string=w438) -> (unsigned byte array=w436:u8[])
        n267 = local write "Picture size"(w452) -> ()
        n268 = local write "Picture size 2"(w453) -> ()
        n269 = Divide(x=w452, y=w448) -> (x/y=w460:dbl)
        n270 = Divide(x=w453, y=w448) -> (x/y=w461:dbl)
        n271 = Array Size(array=w436) -> (size(s)=w435:i32)
        n272 = Subtract(x=w436, y=48) -> (x-y=w442:i32[])
        n273 = Round Toward +Infinity(x=w460) -> (ceil(x): smallest int >= x=→"x":dbl)
        n274 = Round Toward +Infinity(x=w461) -> (ceil(x): smallest int >= x=→"y":dbl)
        n275 = Initialize Array(4, w435) -> (w446:i32[])
        n276 = Initialize Array(1, w435) -> (w444:i32[])
        n277 = In Range and Coerce(upper limit=w446, x=w442, lower limit=w444) -> (coerced(x)=w439:i32[])  [unwired: 1 out]
        n278 = Add(x=w439, y=48) -> (x+y=w441:i32[])
        n279 = Byte Array To String(unsigned byte array=w441) -> (string=w437:string)
        n280 = while {
          shift-right: [w466] -> w434
          shift-left: w437 -> [w470]
          i -> [w462]
          stop <- w465 stop-if-true
          n281 = Increment(x=w462) -> (x+1=w463:i32)
          n282 = String Subset(string=w470, offset (0)=w462, length (rest)=1) -> (substring=w468:string)
          n283 = Search and Replace String(replace all?=TRUE, input string=w470, search string=w468, offset=w463) -> (result string=w466:string)  [unwired: 4 in, 3 out]
          n284 = String Length(string=w466) -> (length=w464:i32)
          n285 = Less?(x=w464, y=w462) -> (x < y?=w465:bool)
        }
        n286 = local write "Laser  Profile"(w434) -> ()
      }
      event "SCANNER EMERGENCY": Value Change {
        n287 = event-data() -> ()  [unwired: 1 in, 5 out]
        n288 = local read "PI SystemNumber"() -> (w473:i32)
        n289 = call "PI Write GPIB.vi"("System no."=w473, "String to send"="0RT", "error in"=w472) -> ("error out"=w475:errorcluster)  [unwired: 16 in]
        n290 = flat-sequence {
          tunnel: [w476] -> w471
          tunnel: w475 -> [w476]
          frame #0 {
            n291 = One Button Dialog(message="Emergency scanner stop appeared!!!\nCheck scanner settings before continue!!!") -> ()  [unwired: 2 out]
          }
        }
      }
      event "SET CCD": Value Change {
        n292 = event-data() -> ()  [unwired: 1 in, 6 out]
        n293 = call "Camera CCD Chip settings"("error in (no error)"=w479) -> ("Horizontal Binning"=w480:dbl, "Vertical Binning"=w485:dbl, "CCD Chip Horizontal Start"=w484:dbl, "CCD Chip Horizontal End"=w482:dbl, "CCD Chip Vertical Start"=w483:dbl, "CCD Chip Vertical End"=w481:dbl, "OK"=w486:bool, "error out"=w478:errorcluster)  [unwired: 11 in]
        n294 = case shown="True" w486 {
          tunnel: w485 -> [_ w494]
          tunnel: w484 -> [_ w493]
          tunnel: w483 -> [_ w492]
          tunnel: w482 -> [_ w491]
          tunnel: w481 -> [_ w490]
          tunnel: w480 -> [_ w489]
          tunnel: [_ w488] -> _
          tunnel: w478 -> [_ w487]
          frame False {
          }
          frame True {
            n295 = flat-sequence {
              tunnel: w494 -> [w501]
              tunnel: w493 -> [w495]
              tunnel: w492 -> [w500]
              tunnel: w491 -> [w499]
              tunnel: w490 -> [w498]
              tunnel: w489 -> [w497]
              tunnel: [w496] -> w488
              tunnel: w487 -> [w496]
              frame #0 {
                n296 = global write "GlobalSetGetConfigureCamera.vi" "Vbin"(w501) -> ()
                n297 = global write "GlobalSetGetConfigureCamera.vi" "Hbin"(w497) -> ()
                n298 = global write "ccdChipPixels.vi" "CCD Chip Vertical Start"(w500) -> ()
                n299 = global write "ccdChipPixels.vi" "CCD Chip horizontal end"(w499) -> ()
                n300 = global write "ccdChipPixels.vi" "CCD Chip Vertical end"(w498) -> ()
                n301 = global write "ccdChipPixels.vi" "CCD Chip horizontal start"(w495) -> ()
                n302 = Subtract(x=w499, y=w495) -> (x-y=w503:dbl)
                n303 = Subtract(x=w498, y=w500) -> (x-y=w502:dbl)
                n304 = Increment(x=w503) -> (x+1=w505:dbl)
                n305 = Increment(x=w502) -> (x+1=w504:dbl)
                n306 = Multiply(x=w505, y=w504) -> (x*y=w506:dbl)
                n307 = global write "ccdChipPixels.vi" "CCD Chip Size"(w506) -> ()
              }
            }
          }
        }
      }
      event "Set Temperature": Value Change {
        n308 = event-data() -> ()  [unwired: 1 in, 6 out]
        n309 = call "camera cooling"("error in (no error)"=w508) -> ("Temperature"=w509:dbl, "OK"=w510:bool, "error out"=w507:errorcluster)  [unwired: 16 in]
        n310 = case shown="True" w510 {
          tunnel: w509 -> [_ w514]
          tunnel: w507 -> [w511 w513]
          tunnel: [w511 w512] -> _
          frame False {
          }
          frame True {
            n311 = call "CheckTemperature.vi"("error in (no error)"=w513, "temperature in"=w514) -> ("error out"=w512:errorcluster)  [unwired: 9 in]
          }
        }
      }
      event "Cam (Defocused)": Value Change {
        n312 = event-data() -> ()  [unwired: 1 in, 6 out]
        n313 = global write "CamDef.vi" "CamDef"(w515) -> ()
      }
      event "OPEN SHUTER": Value Change {
        n314 = event-data() -> ()  [unwired: 1 in, 6 out]
        n315 = case shown="False" w517 {
          tunnel: [Shutter_mode_typedef."Close" ("mode") Shutter_mode_typedef."Open" ("mode")] -> w521
          tunnel: w518 -> [w523 w524]
          tunnel: [w523 w524] -> w520
          frame False {
          }
          frame True {
          }
        }
        n316 = call "SetShutter.vi"("type"=Shutter_type_typedef."TTL Low", "mode"=w521, "error in (no error)"=w520) -> ("error out"=w516:errorcluster)  [unwired: 11 in, 1 out]
      }
      event "Close": Value Change {
        n317 = event-data() -> ()  [unwired: 1 in, 6 out]
        n318 = case shown="True" w526 {
          tunnel: [Shutter_mode_typedef."Open" ("mode") Shutter_mode_typedef."Open" ("mode")] -> w530
          tunnel: w527 -> [w532 w533]
          tunnel: [w532 w533] -> w529
          frame False {
          }
          frame True {
          }
        }
        n319 = call "SetShutter.vi"("type"=Shutter_type_typedef."TTL Low", "mode"=w530, "error in (no error)"=w529) -> ()  [unwired: 11 in, 2 out]
      }
      event "Exposure": Value Change {
        n320 = event-data() -> ()  [unwired: 1 in, 6 out]
        n321 = call "Camera kinetic settings"("error in (no error)"=w538) -> ("Exposure time"=w535:dbl, "OK"=w536:bool, "error out"=w537:errorcluster)  [unwired: 16 in]
        n322 = case shown="True" w536 {
          tunnel: w535 -> [_ w539]
          frame False {
          }
          frame True {
            n323 = global write "GlobalSetGetConfigureCamera.vi" "Exposure"(w539) -> ()
          }
        }
      }
      event "Gain": Value Change {
        n324 = event-data() -> ()  [unwired: 1 in, 6 out]
        n325 = call "set gain"("error in (no error)"=w540) -> ("gain"=w542:dbl, "OK"=w541:bool)  [unwired: 16 in, 1 out]
        n326 = case shown="True" w541 {
          tunnel: w542 -> [_ w543]
          frame False {
          }
          frame True {
            n327 = global write "GlobalSetGetConfigureCamera.vi" "gain"(w543) -> ()
          }
        }
      }
      event "Start": Value Change {
        n328 = event-data() -> ()  [unwired: 1 in, 6 out]
        n329 = global write "GetPicture.vi" "GetPicture"(TRUE ("GetPicture")) -> ()
      }
      event "Measurement Time": Value Change {
        n330 = event-data() -> ()  [unwired: 1 in, 6 out]
        n331 = global write "GlobalSetGetConfigureCamera.vi" "Exposure"(w545) -> ()
      }
      event "Stop": Value Change {
        n332 = event-data() -> ()  [unwired: 1 in, 6 out]
        n333 = global write "StopGetPic.vi" "Stop"(TRUE ("Stop")) -> ()
      }
      event "Stop Program": Value Change {
        n334 = event-data() -> ()  [unwired: 1 in, 6 out]
        n335 = flat-sequence {
          tunnel: w547 -> [w551]
          tunnel: [w551] -> w550
          frame #0 {
            n336 = local write "Global Stop"(TRUE ("Global Stop")) -> ()
          }
        }
        n337 = local read "PI SystemNumber"() -> (w549:i32)
        n338 = call "Close connection if open.vi"("System no."=w549, "error in"=w550) -> ("error out"=w548:errorcluster)  [unwired: 16 in, 1 out]
      }
    }
    "z-position" <- w104
    "y-position" <- w88
    "x-position" <- w103
  }
  n339 = while {
    shift-right: [w559] -> w10
    shift-left: w6 -> [w556]
    shift-right: [w561] -> _
    shift-left: w6 -> [w566]
    tunnel: w18 -> [w560]
    tunnel: "Image Measurent Parameters" -> [w555]
    tunnel: [w554] -> _
    tunnel: "Sample description" -> [w553]
    stop <- w564 stop-if-true
    n340 = case shown="No Error" w556 {
      selector: w556 -> [w572 w1445]
      tunnel: w566 -> [w582 w1447]
      tunnel: [w581 TRUE ("Global Stop")] -> w563
      tunnel: [w577 w1447] -> w562
      tunnel: w560 -> [w576 _]
      tunnel: [w575 w1445] -> w559
      tunnel: [w573 T25."No Measurement" ("Do Measurement")] -> w557
      tunnel: w555 -> [w570 _]
      tunnel: [w569 w1445] -> w554
      tunnel: w553 -> [w567 _]
      frame No Error {
        n341 = while {
          shift-right: [w1443] -> w578
          shift-left: w582 -> [w1443]
          tunnel: [w1438] -> w580
          tunnel: [w1440] -> w579
          tunnel: [w1439] -> w574
          stop <- w1444 stop-if-true
          w1439 = FALSE ("FiFo Overrun")
          # "Wait for Start"
          n342 = local read "Task"() -> (w1438:T10)
          n343 = local read "Global Stop"() -> (w1440:bool)
          n344 = Wait (ms)(milliseconds to wait=u32 100) -> ()  [unwired: 1 out]
          n345 = local write "Stop Measurement"(w1439) -> ()
          n346 = Greater Than 0?(x=w1438) -> (x > 0?=w1442:bool)
          n347 = Or(x=w1442, y=w1440) -> (x .or. y?=w1444:bool)
        }
        n348 = control-ref of="WS File Tree"() -> (w571:refnum<vi>)
        n349 = case shown="\"Find Single Mol.\"" w580 {
          selector: w580 -> [_ _ w948 _ _ _]
          tunnel: w572 -> [w583 w631 w856 w1130 w1199 w1401]
          tunnel: [w583 w601 w904 w1119 w1197 w1401] -> w575
          tunnel: [w584 FALSE ("Global Stop") FALSE ("Global Stop") FALSE ("Global Stop") FALSE ("Global Stop") FALSE ("Global Stop")] -> w581
          tunnel: w579 -> [w584 _ _ _ _ _]
          tunnel: w578 -> [w586 w615 w855 w1129 w1198 w1402]
          tunnel: [w586 w615 w969 w1129 w1198 w1400] -> w577
          tunnel: w576 -> [_ w681 w906 _ _ _]
          tunnel: [T25."No Measurement" ("Do Measurement") T25."No Measurement" ("Do Measurement") w947 T25."No Measurement" ("Do Measurement") T14."No Measurement" ("Do Measurement") w1399] -> w573
          tunnel: w571 -> [_ _ w937 _ _ _]
          tunnel: w570 -> [_ w659 _ _ _ _]
          tunnel: [w583 w633 w930 w1119 _ _] -> w569
          tunnel: "Laser pulse duration" -> [_ _ w912 _ _ _]
          tunnel: w567 -> [_ _ w903 _ _ _]
          frame "No Measurement", Default {
          }
          frame "Aquire Image" {
            w594 = 200
            w625 = T33."Image File" ("Measurement Type")
            w662 = 32768 ("dimension size")
            # "TODO:\n- FIFO Read Flag Buffer Half Full?\n- auto square pixels"
            # "Image Intensity Array"
            n350 = Index Array(array=w681) -> (element=w680:T34)  [unwired: 1 in]
            n351 = Unbundle By Name(w680) -> ("Dev"=w653:i32)
            n352 = local read "PI SystemNumber"() -> (w603:i32)
            n353 = Index Array(array=string[] ["yx", "yz", "xy", "xz", "zy", "zx"] ("Array"), index="Axis") -> (element=w608:string)
            n354 = stacked-sequence {
              seq-local: [w693 _] -> [_ w720]
              seq-local: [w692 _] -> [_ w721]
              seq-local: [w691 _] -> [_ w716]
              seq-local: [w687 _] -> [_ w714]
              seq-local: [w686 _] -> [_ w713]
              seq-local: [w685 _] -> [_ w712]
              seq-local: [w688 _] -> [_ w708]
              tunnel: "Picture size" -> [w706 _]
              tunnel: "Picture size 2" -> [w705 _]
              tunnel: w659 -> [w704 _]
              tunnel: "X-Position" -> [w703 _]
              tunnel: "Y-Position" -> [w702 _]
              tunnel: "Z-Position" -> [w701 _]
              tunnel: "Axis" -> [w695 _]
              tunnel: "Resolution" -> [w691 _]
              tunnel: [w694 _] -> w587
              tunnel: [_ w722] -> w632
              tunnel: w631 -> [w689 _]
              tunnel: w608 -> [_ w719]
              tunnel: "Laser  Profile" -> [_ w718]
              tunnel: "Pixel time" -> [w690 w717]
              tunnel: w603 -> [_ w715]
              tunnel: [_ w707] -> w628
              tunnel: [_ w711] -> w627
              tunnel: [_ w710] -> w626
              tunnel: [_ w709] -> w618
              frame #0 {
                n355 = call "PI_CheckScan.vi"("Picture size"=w706, "Picture size 2"=w705, "Axis"=w695, "x-Position"=w703, "y-Position"=w702, "z-Position"=w701, "error in (no error)"=w689) -> ("error out"=w688:errorcluster, "Picture size out"=w692:dbl, "Picture size out 2"=w693:dbl, "a0"=w687:dbl, "b0"=w686:dbl, "c0"=w685:dbl)  [unwired: 7 in]
                n356 = Divide(x=w692, y=w691) -> (x/y=w698:dbl)
                n357 = Divide(x=w693, y=w691) -> (x/y=w699:dbl)
                n358 = local write "Picture size 2"(w693) -> ()
                n359 = local write "Picture size"(w692) -> ()
                n360 = Round Toward +Infinity(x=w698) -> (ceil(x): smallest int >= x=w697:dbl)
                n361 = Round Toward +Infinity(x=w699) -> (ceil(x): smallest int >= x=w696:dbl)
                n362 = Bundle("a0"=w687, "b0"=w686, "c0"=w685) -> (w700:cluster{"a0":dbl, "b0":dbl, "c0":dbl})  [unwired: 1 in]
                n363 = Bundle By Name(cluster=w704, "Position"=w700, "Axis 1 Pixels"=w697, "Axis 2 Pixels"=w696, "Axis"=w695, "Resolution"=w691, "PixelTime"=w690) -> (w694:T8)
              }
              frame #1 {
                n364 = call "PI_AreaScan_Prepare_1.vi"("System"=w715, "Laser"=w718, "Axis"=w719, "da"=w721, "db"=w720, "error in (no error)"=w708, "a0"=w714, "b0"=w713, "Resolution"=w716, "c0"=w712, "Pixel time"=w717) -> ("Tacq"=w707:dbl, "lp"=w710:i32, "ap"=w711:i32, "Trigger"=w709:dbl[], "error out"=w722:errorcluster)  [unwired: 4 in]
                "Measure. time" <- w707
              }
            }
            n365 = String To Byte Array(string="Laser  Profile") -> (unsigned byte array=w610:u8[])
            n366 = Unbundle By Name(w587) -> ("Axis 1 Pixels"=w640:dbl, "Axis 2 Pixels"=w641:dbl, "Resolution"=w638:dbl, "PixelTime"=w622:dbl)  [unwired: 2 out]
            n367 = control-ref of="WS File Tree"() -> (w665:refnum<vi>)
            n368 = local read "Workspace"() -> (w670:path)
            n369 = Divide(x=w640, y=w638) -> (x/y=w649:dbl)
            n370 = Divide(x=w641, y=w638) -> (x/y=w651:dbl)
            n371 = call "HH_Set.vi"("Device List"=w681, "CFD Settings"="CFD Settings", "error in (no error)"=w632, "SyncDiv"=8) -> ("ht3 header out"=w645:T35, "Sync Rate"=w643:i32, "error out"=w617:errorcluster)  [unwired: 7 in, 2 out]
            n372 = Divide(x=w622, y=1000) -> (x/y=w620:dbl)
            n373 = control-ref of="Image"() -> (w647:refnum<vi>)
            n374 = Round Toward +Infinity(x=w649) -> (ceil(x): smallest int >= x=w648:dbl)
            n375 = Round Toward +Infinity(x=w651) -> (ceil(x): smallest int >= x=w650:dbl)
            n376 = call "MTS_PreapareImage.vi"("WS File Tree"=w665, "Workspace"=w670, "Measurement Type"=w625, "Image Measurent Parameters"=w587, "error in"=w617, "Trigger"=w618) -> ("File Name (dup)"=w655:path, "File No"=→"Last Image File No":i32, "Image Header"=w657:T36, "Comment"=w658:string, "error out"=w616:errorcluster)  [unwired: 5 in]
            n377 = Divide(x=1024, y=w643) -> (x/y=w624:dbl)
            n378 = local write "Active pt3"(w655) -> ()
            n379 = Multiply(x=w628, y=1000) -> (x*y=w637:dbl)
            n380 = call "Scan_SetGraphScales.vi"("error in (no error)"=w616, "Image Measurent Parameters"=w587, "Image"=w647) -> ("error out"=w646:errorcluster)  [unwired: 8 in]
            n381 = Subtract(x=w610, y=48) -> (x-y=w609:i32[])
            n382 = Initialize Array(0 ("element"), w648, w650) -> (w621:i32[][])
            n383 = Initialize Array(0, 5, 2) -> (w607:i32[][])
            n384 = Replace Array Subset(array=w607, new element=w609, index (col)=0) -> (w605:i32[][])  [unwired: 1 in]
            n385 = call "HT3_Create.vi"("Laser"=w605, "Image Header in"=w657, "Save pt3"="Save Files", "Measurement Type"=w625, "error in"=w646, "Comment"=w658, "ht3 Header in"=w645, "File Path"=w655) -> ("error out"=w671:errorcluster, "FileHeaderPos"=w661:T37, "refnum out"=w669:refnum<file>)  [unwired: 1 in]
            n386 = Round Toward +Infinity(x=w637) -> (ceil(x): smallest int >= x=w635:dbl)
            n387 = call "HH_Start.vi"("Device Index"=w653, "Acq. Time"=w635, "error in (no error)"=w671) -> ("error out"=w678:errorcluster)  [unwired: 11 in, 1 out]
            n388 = Unbundle By Name(w678) -> ("status"=w679:bool)
            n389 = Not(x=w679) -> (.not. x?=w677:bool)
            n390 = Initialize Array(u32 0, w662) -> (w674:u32[])
            n391 = case shown="True" w677 {
              tunnel: [w770 w801] -> w676
              tunnel: w603 -> [_ w796]
              tunnel: w678 -> [w771 w797]
              tunnel: w653 -> [w769 w788]
              tunnel: w621 -> [_ w773]
              tunnel: w674 -> [_ w795]
              tunnel: w662 -> [_ w794]
              tunnel: [w768 w793] -> w673
              tunnel: [w768 w792] -> w672
              tunnel: w669 -> [w767 w791]
              tunnel: [w767 w790] -> w668
              tunnel: [0 ("Num Records Total") w789] -> w667
              tunnel: [0.0 w782] -> w666
              tunnel: w608 -> [_ w785]
              tunnel: [dbl[] [] w779] -> w623
              tunnel: w620 -> [_ w775]
              tunnel: w618 -> [_ w774]
              frame False {
                (unwired) i32[][] [] ("Image Array Out")
                (unwired) u64[] [] ("Histograms")
                w768 = FALSE ("Stop Measurement")
                n392 = call "HH_Stop.vi"("Device Index"=w769, "error in (no error)"=w771) -> ("error out"=w770:errorcluster)  [unwired: 12 in, 1 out]
              }
              frame True {
                # "Overflow Interv. Time (s)"
                # "No Error"
                n393 = call "PI Start WG.vi"("System no."=w796, "axis"=w785, "Generator"=T26."both axis", "Init DDL"=T27."none", "increment"=T27."slow axis", "error in"=w797, "saved data"=T28."actual position") -> ("error out"=w798:errorcluster)  [unwired: 12 in]
                n394 = Initialize Array(0, 5) -> (w776:i32[])
                n395 = while {
                  tunnel: w788 -> [w821]
                  tunnel: w795 -> [w837]
                  tunnel: w794 -> [w836]
                  shift-right: [w822] -> w800
                  shift-left: w798 -> [w838]
                  shift-right: [FALSE ("Reset")] -> _
                  shift-left: TRUE ("Reset") -> [w809]
                  tunnel: [w830] -> w793
                  tunnel: [w826] -> w792
                  tunnel: w791 -> [w828]
                  tunnel: [w827] -> w790
                  tunnel: [w805] -> w789
                  tunnel: [w804] -> w782
                  shift-right: [w818] -> w781
                  shift-left: w776 -> [w816]
                  tunnel: [w815] -> w780
                  tunnel: w775 -> [w812]
                  tunnel: w774 -> [_]
                  shift-right: [w803] -> w772
                  shift-left: w773 -> [w811]
                  i -> [w814]
                  stop <- w835 stop-if-true
                  n396 = call "HH_FIFORead.vi"("Device Index"=w821, "Buffer In"=w837, "Count"=w836, "error in (no error)"=w838) -> ("OK"=w831:bool, "Buffer Out"=w808:u32[], "Data Count"=w807:i32, "FiFo Overrun"=w830:bool, "error out"=w829:errorcluster)  [unwired: 7 in]
                  n397 = local write "Buffer Overrun"(w830) -> ()
                  n398 = Unbundle(w829) -> ("status"=w834:bool)  [unwired: 2 out]
                  n399 = call "HT3_Write.vi"("error in"=w829, "Data Count"=w807, "Data in"=w808, "refnum in"=w828) -> ("error out"=w823:errorcluster, "refnum out"=w827:refnum<file>)  [unwired: 6 in]
                  n400 = call "GetCountRates.vi"("error in (no error)"=w823, "DeviceIndex"=w821) -> ("error out"=w822:errorcluster, "CntRates"=w820:dbl[], "SyncRate"=w813:i32)  [unwired: 1 in]
                  n401 = local read "Stop Measurement"() -> (w825:bool)
                  n402 = local read "Global Stop"() -> (w824:bool)
                  n403 = Multiply(x=w812, y=w813) -> (x*y=w802:dbl)
                  n404 = Compound Arithmetic op=OR(invert w831, w834, w824, w825) -> (w835:bool)
                  n405 = Insert Into Array(array=w820, index=0, new element=w813) -> (w817:dbl[])
                  n406 = call "HH_ToImage.vi"("Data In"=w808, "Reset"=w809, "Image Array In"=w811, "Data Count"=w807, "Pixel Time (Laser Pulses)"=w802) -> ("Image Array Out"=w803:i32[][], "Histograms"=→"Histogram":i32[][], "Total Oveflow Count"=w804:u64, "Num Records Total"=w805:i64, "Traces"=→"Trace":i32[][])  [unwired: 4 in, 2 out]
                  n407 = Or(x=w825, y=w824) -> (x .or. y?=w826:bool)
                  n408 = Add(x=w816, y=w817) -> (x+y=w818:dbl[])
                  n409 = Wait (ms)(milliseconds to wait=u32 2) -> ()  [unwired: 1 out]
                  n410 = Increment(x=w814) -> (x+1=w815:i32)
                }
                "Image" <- w772
                n411 = call "HH_Stop.vi"("Device Index"=w788, "error in (no error)"=w800) -> ("error out"=w801:errorcluster)  [unwired: 12 in, 1 out]
                n412 = Divide(x=w781, y=w780) -> (x/y=w779:dbl[])
              }
            }
            n413 = flat-sequence {
              tunnel: w676 -> [w741]
              tunnel: [w730] -> w602
              tunnel: w673 -> [w743]
              tunnel: w672 -> [w732]
              tunnel: w603 -> [w740]
              tunnel: [w739] -> w600
              tunnel: w668 -> [w737]
              tunnel: w667 -> [w736]
              tunnel: w666 -> [w726]
              tunnel: w661 -> [w731]
              tunnel: w624 -> [w727]
              tunnel: w623 -> [w723]
              frame #0 {
                # "Count Rate (per s)"
                # "Finish after Aquire Image"
                n414 = Multiply(x=w727, y=w726) -> (x*y=w725:dbl)
                n415 = Or(x=w732, y=w743) -> (x .or. y?=w742:bool)
                n416 = case shown="False" w742 {
                  tunnel: w741 -> [w748 w758]
                  tunnel: w740 -> [w746 w759]
                  tunnel: [w745 w759] -> w739
                  tunnel: [w747 w757] -> w738
                  tunnel: [enum16{"timeover", "manual", "overflow"}."timeover" ("Stop Reason") w762] -> w733
                  tunnel: w732 -> [w744 w760]
                  frame False {
                    # "Stop WaveGen\nif Aborted"
                    n417 = case shown="True" w744 {
                      tunnel: w748 -> [w750 w755]
                      tunnel: [w750 w754] -> w747
                      tunnel: w746 -> [w751 w753]
                      tunnel: [w751 w753] -> w745
                      frame False {
                      }
                      frame True {
                        n418 = call "PI Write GPIB.vi"("System no."=w753, "String to send"="0RT", "error in"=w755) -> ("error out"=w754:errorcluster)  [unwired: 16 in]
                      }
                    }
                  }
                  frame True {
                    n419 = Select(t=enum16{"timeover", "manual", "overflow"}."manual" ("Stop Reason"), s=w760, f=enum16{"timeover", "manual", "overflow"}."overflow" ("Stop Reason")) -> (s? t:f=w762:enum16{"timeover", "manual", "overflow"})
                    n420 = call "PI Write GPIB.vi"("System no."=w759, "String to send"="0RT", "error in"=w758) -> ("error out"=w757:errorcluster)  [unwired: 16 in]
                  }
                }
                n421 = Multiply(x=w725, y=1000.0) -> (x*y=w735:dbl)
                n422 = property on="Aquire Image" class="Bool"("BoolText.Text"="Aquire Image" ("Caption.Text"), "BoolText.TextColor"=u32 0 ("Boolean Text.Colors:FG Color")) -> ()  [unwired: 2 in, 2 out]
                n423 = To Long Integer(number=w735) -> (32bit integer=w734:i32)
                n424 = call "HT3_Finish.vi"("FileHeaderPos"=w731, "Rates"=w723, "Stop Reason"=w733, "error in"=w738, "Num Records"=w736, "Stop After (ms)"=w734, "refnum in"=w737) -> ("error out"=w730:errorcluster)  [unwired: 4 in]
              }
            }
            n425 = local read "X-Position"() -> (w593:dbl)
            n426 = local read "Y-Position"() -> (w592:dbl)
            n427 = local read "Z-Position"() -> (w591:dbl)
            n428 = Subtract(x=w594, y=w593) -> (x-y=w590:dbl)
            n429 = Subtract(x=w594, y=w592) -> (x-y=w589:dbl)
            n430 = Subtract(x=w594, y=w591) -> (x-y=w588:dbl)
            n431 = global read "GlobalConAxisPI.vi" "Conn. Axes"() -> (w599:string[])
            n432 = call "AOTF-Trigger_1.vi"("Channel"="Laser  Profile", "error in (no error)"=w632, "Triggered"=TRUE, "lp"=w626, "ap"=w627) -> ("error out"=w633:errorcluster)  [unwired: 2 in]
            n433 = Build Array(w590, w589, w588) -> (w598:dbl[])
            n434 = call "MOV.vi"("System no."=w600, "Axes to move"=w599, "Position values"=w598, "error in"=w602) -> ("error out"=w601:errorcluster)  [unwired: 15 in]
          }
          frame "Point Measurement", "Auto Point" {
            w874 = 200
            w879 = 200
            w907 = 0
            w935 = 32768 ("dimension size")
            n435 = Index Array(array=w906) -> (element=w973:T34)  [unwired: 1 in]
            n436 = Unbundle By Name(w973) -> ("Dev"=w892:i32)
            n437 = Equal?(x=w948, y=T10."Auto Point" ("Task")) -> (x = y?=w844:bool)
            n438 = local read "concatenated string"() -> (w899:string)
            n439 = And(x=w844, y="Autopoint-Autofocus Z") -> (x .and. y?=w936:bool)
            n440 = Or(x="Point Defocussed Cam", y="Auto Defocussed Cam") -> (x .or. y?=w861:bool)
            n441 = Select(t="Auto Measurement Time (ms)", s=w844, f="Measurement Time") -> (s? t:f=w845:i32)
            n442 = local read "X-Position"() -> (w954:dbl)
            n443 = local read "Y-Position"() -> (w953:dbl)
            n444 = local read "Z-Position"() -> (w889:dbl)
            n445 = Select(t="AutoPoint" ("Measurement Type"), s=w844, f="Point" ("Measurement Type")) -> (s? t:f=w898:string)
            n446 = case shown="True" w861 {
              tunnel: [w975 w980] -> w854
              tunnel: w855 -> [w975 w981]
              tunnel: w845 -> [_ w978]
              frame False {
              }
              frame True {
                n447 = global read "GlobalSetGetConfigureCamera.vi" "Exposure"() -> (w976:sgl)
                n448 = Greater?(x=w976, y=w978) -> (0:w979:bool)
                n449 = case shown="False" w979 {
                  tunnel: w978 -> [_ w983]
                  tunnel: [w982 w983] -> w977
                  tunnel: w976 -> [w982 _]
                  frame False {
                  }
                  frame True {
                  }
                }
                n450 = call "PrepCamera.vi"("mesTime"=w977, "error out 2"=w981) -> ("error out"=w980:errorcluster)  [unwired: 25 in]
              }
            }
            n451 = Select(t=T10."Auto Measurement Control" ("Task"), s=w844, f=T25."No Measurement" ("Do Measurement")) -> (s? t:f=w947:T10)
            n452 = local read "NxtAutMesPoint"() -> (w893:i32)
            n453 = Multiply(x=w845, y=1000) -> (x*y=w846:i32)
            n454 = local read "Pattern"() -> (w894:dbl[][])
            n455 = Concatenate Strings(w899, w898) -> (w897:string)
            n456 = Bundle("X-Position"=w954, "Y-Position"=w953, "Z-Position"=w889) -> (w938:T38)  [unwired: 1 in]
            n457 = call "MTS_AutoPointCords.vi"("Is Auto Point"=w844, "Cords In"=w938, "Next Auto Measure Point"=w893, "Pattern"=w894) -> ("Cords"=w925:T38)  [unwired: 7 in]
            n458 = Unbundle By Name(w925) -> ("X-Position"=w865:dbl, "Y-Position"=w866:dbl, "Z-Position"=w875:dbl)
            n459 = Subtract(x=w879, y=w866) -> (x-y=w878:dbl)
            n460 = Subtract(x=w879, y=w865) -> (x-y=w877:dbl)
            n461 = Subtract(x=w879, y=w875) -> (x-y=w876:dbl)
            n462 = local read "PI SystemNumber"() -> (w887:i32)
            n463 = global read "GlobalConAxisPI.vi" "Conn. Axes"() -> (w881:string[])
            n464 = Build Array(w878, w877, w876) -> (w880:dbl[])
            n465 = local read "Last Image File No"() -> (w941:i32)
            n466 = call "MOV.vi"("System no."=w887, "Axes to move"=w881, "Position values"=w880, "No.of digits"=i16 3, "error in"=w856) -> ("error out"=w869:errorcluster)  [unwired: 14 in]
            n467 = flat-sequence {
              tunnel: w869 -> [w984]
              tunnel: [w984] -> w868
              frame #0 {
                n468 = Wait (ms)(milliseconds to wait=u32 100) -> ()  [unwired: 1 out]
              }
            }
            n469 = Select(t=T29."Auto Point" ("Measurement Type"), s=w844, f=T29."Point Measurement" ("Measurement Type")) -> (s? t:f=w942:T29)
            n470 = Select(t=w941, s=w844, f=-1) -> (s? t:f=w939:i32)
            n471 = local read "Workspace"() -> (w963:path)
            n472 = call "MTS_GenFileComment.vi"("Measurement Type"=w942, "Parent File No"=w939, "Info"=w903, "Upper Left"=w925, "error in"=w854) -> ("Comment"=w964:string, "error out"=w962:errorcluster)  [unwired: 7 in, 2 out]
            n473 = Not(x="Adjustment") -> (.not. x?=w901:bool)
            n474 = call "MTS_GetNextFileName.vi"("error in (no error)"=w962, "File Type"="ht3", "Measurement Type"=w897, "Workspace"=w963) -> ("error out"=w957:errorcluster, "Next File Name"=w956:path)  [unwired: 6 in]
            n475 = local read "CFD Settings"() -> (w932:T7)
            n476 = case shown="True" w901 {
              tunnel: w957 -> [w998 w1006]
              tunnel: w956 -> [_ w1005]
              tunnel: [w998 w1004] -> w857
              tunnel: [path "D:/tmp.ht3" w999] -> w955
              tunnel: w942 -> [_ w1001]
              tunnel: w939 -> [_ w1003]
              tunnel: w937 -> [_ w1000]
              frame False {
              }
              frame True {
                n477 = call "MTS_AddFileToWorkspace.vi"("File Name"=w1005, "File Type"=T30."pt3 File", "Measurement Type"=w1001, "error in (no error)"=w1006, "Parent"=w1003, "Tree Refnum"=w1000) -> ("File Name (dup)"=w999:path, "error out"=w1004:errorcluster)  [unwired: 7 in, 1 out]
              }
            }
            n478 = call "POS?.vi"("System no."=w887, "Axes to query"=w881, "All axes?"=TRUE, "error in"=w868) -> ("Position"=w885:dbl[], "error out"=w888:errorcluster)  [unwired: 14 in]
            n479 = call "HH_Set.vi"("Device List"=w906, "CFD Settings"=w932, "error in (no error)"=w888) -> ("ht3 header out"=w952:T35, "Sync Rate"=w922:i32, "error out"=w950:errorcluster)  [unwired: 8 in, 2 out]
            n480 = Index Array(array=w885, index #1=0 ("index"), index #2=1 ("index"), index #3=2 ("index")) -> (element #1=w873:dbl, element #2=w872:dbl, element #3=w871:dbl)
            n481 = Bundle By Name(cluster=w952, "AcquisitionTime (ms)"=w846) -> (w951:T35)
            n482 = Divide(x=65536 ("n"), y=w922) -> (x/y=w923:dbl)
            n483 = Subtract(x=w874, y=w873) -> (x-y=w843:dbl)
            n484 = Subtract(x=w874, y=w871) -> (x-y=w870:dbl)
            n485 = Subtract(x=w874, y=w872) -> (x-y=w842:dbl)
            n486 = property on="y-position" class="DigNum (strict)"("Value"=w843) -> ()  [unwired: 2 in, 2 out]
            n487 = property on="z-position" class="DigNum (strict)"("Value"=w870) -> ()  [unwired: 2 in, 2 out]
            n488 = case shown="True" w936 {
              tunnel: w950 -> [w1007 w1015]
              tunnel: [w1007 w1014] -> w949
              tunnel: w887 -> [_ w1009]
              tunnel: w923 -> [_ w1013]
              tunnel: w925 -> [_ w1012]
              tunnel: w892 -> [_ w1008]
              frame False {
              }
              frame True {
                # "Auto Z"
                n489 = call "MTS_AutoZPos.vi"("PH Dev"=w1008, "OFlow Interv [s]"=w1013, "PI System no."=w1009, "error in"=w1015, "Start Point"=w1012) -> ("New Z"=w1011:dbl, "Counts"=→"Counts":u32[], "error out"=w1014:errorcluster)  [unwired: 7 in, 1 out]
                n490 = local write "Z-Position"(w1011) -> ()
              }
            }
            n491 = property on="x-position" class="DigNum (strict)"("Value"=w842) -> ()  [unwired: 2 in, 2 out]
            n492 = Initialize Array(u32 0, w935) -> (w967:u32[])
            n493 = global read "ccdChipPixels.vi" "CCD Chip horizontal start"() -> (w852:i32)
            n494 = global read "ccdChipPixels.vi" "CCD Chip horizontal end"() -> (w853:i32)
            n495 = global read "ccdChipPixels.vi" "CCD Chip Vertical Start"() -> (w850:i32)
            n496 = global read "ccdChipPixels.vi" "CCD Chip Vertical end"() -> (w851:i32)
            n497 = Subtract(x=w853, y=w852) -> (x-y=w848:i32)
            n498 = Subtract(x=w851, y=w850) -> (x-y=w847:i32)
            n499 = flat-sequence {
              tunnel: w970 -> [w1019]
              tunnel: w858 -> [w1036]
              tunnel: [w1017] -> w969
              tunnel: [w1033] -> w905
              tunnel: w966 -> [w1038]
              tunnel: w965 -> [w1029]
              tunnel: w959 -> [w1032]
              tunnel: w958 -> [w1031]
              tunnel: w934 -> [w1028]
              tunnel: w927 -> [w1025]
              tunnel: w926 -> [w1024]
              tunnel: w861 -> [w1016]
              frame #0 {
                # "Finish after Measurement"
                n500 = case shown="False" w1016 {
                  tunnel: w1019 -> [w1040 w1045]
                  tunnel: [w1040 w1042] -> w1018
                  frame False {
                  }
                  frame True {
                    n501 = call "SetShutter.vi"("type"=Shutter_type_typedef."TTL High", "mode"=Shutter_mode_typedef."Close", "error in (no error)"=w1045) -> ("error out"=w1047:errorcluster)  [unwired: 11 in, 1 out]
                    n502 = call <vilib>:"Clear Errors.vi"("error in (no error)"=w1047) -> ("error out"=w1046:errorcluster)  [unwired: 6 in]
                    n503 = call "AbortAcquisition.vi"("error in (no error)"=w1046) -> ("error out"=w1041:errorcluster)  [unwired: 1 in, 1 out]
                    n504 = call <vilib>:"Clear Errors.vi"("error in (no error)"=w1041) -> ("error out"=w1042:errorcluster)  [unwired: 6 in]
                  }
                }
                n505 = Or(x=w1029, y=w1038) -> (x .or. y?=w1037:bool)
                n506 = Index Array(array=w1025, index=0) -> (element=w1026:dbl)
                n507 = case shown="False" w1037 {
                  tunnel: w1036 -> [w1049 w1050]
                  tunnel: [w1049 w1050] -> w1034
                  tunnel: [enum16{"timeover", "manual", "overflow"}."timeover" ("Stop Reason") w1053] -> w1030
                  tunnel: w1029 -> [_ w1051]
                  frame False {
                  }
                  frame True {
                    n508 = Select(t=enum16{"timeover", "manual", "overflow"}."manual" ("Stop Reason"), s=w1051, f=enum16{"timeover", "manual", "overflow"}."overflow" ("Stop Reason")) -> (s? t:f=w1053:enum16{"timeover", "manual", "overflow"})
                  }
                }
                n509 = Divide(x=w1024, y=w1026) -> (x/y=w1023:dbl)
                n510 = Multiply(x=1024000, y=w1023) -> (x*y=w1021:dbl)
                n511 = To Long Integer(number=w1021) -> (32bit integer=w1020:i32)
                n512 = property on="Point Measurement" class="Bool"("BoolText.Text"="Point Measurement" ("Caption.Text"), "BoolText.TextColor"=u32 0 ("Boolean Text.Colors:FG Color")) -> ()  [unwired: 2 in, 2 out]
                n513 = call "HT3_Finish.vi"("FileHeaderPos"=w1028, "Rates"=w1025, "Stop Reason"=w1030, "error in"=w1034, "Num Records"=w1031, "Stop After (ms)"=w1020, "refnum in"=w1032) -> ("error out"=w1033:errorcluster)  [unwired: 4 in]
                n514 = Merge Errors(w1019, w1018) -> (w1017:errorcluster)
              }
            }
            n515 = local read "Laser  Profile"() -> (w921:string)
            n516 = String To Byte Array(string=w921) -> (unsigned byte array=w919:u8[])
            n517 = Subtract(x=w919, y=48) -> (x-y=w914:i32[])
            n518 = String Length(string=w921) -> (length=w911:i32)
            n519 = Initialize Array(0, 5, 2) -> (w915:i32[][])
            n520 = Replace Array Subset(array=w915, new element=w914, index (col)=w907) -> (w913:i32[][])  [unwired: 1 in]
            n521 = Array Subset(array=w912, index=w907, length=w911) -> (w910:i32[])
            n522 = Replace Array Subset(array=w913, new element=w910, index (col)=1) -> (w909:i32[][])  [unwired: 1 in]
            n523 = call "HT3_Create.vi"("Laser"=w909, "Save pt3"=w901, "error in"=w949, "Comment"=w964, "ht3 Header in"=w951, "File Path"=w955) -> ("error out"=w890:errorcluster, "FileHeaderPos"=w934:T37, "refnum out"=w960:refnum<file>)  [unwired: 3 in]
            n524 = call "HH_Start.vi"("Device Index"=w892, "Acq. Time"=w846, "error in (no error)"=w890) -> ("error out"=w860:errorcluster)  [unwired: 11 in, 1 out]
            n525 = case shown="True" w861 {
              tunnel: [w986 w990] -> w840
              tunnel: w890 -> [w986 w989]
              tunnel: w844 -> [_ w988]
              tunnel: [_ w987] -> w849
              frame False {
              }
              frame True {
                n526 = control-ref of="NxtAutMesPoint"() -> (w995:refnum<vi>)
                n527 = control-ref of="Workspace"() -> (w996:refnum<vi>)
                n528 = control-ref of="y-position"() -> (w992:refnum<vi>)
                n529 = control-ref of="x-position"() -> (w993:refnum<vi>)
                n530 = control-ref of="z-position"() -> (w991:refnum<vi>)
                n531 = control-ref of="Pattern"() -> (w994:refnum<vi>)
                n532 = call "DefocussedImage.vi"("Path in"=w996, "reference"=w995, "Boolean"=w988, "reference 2"=w994, "reference 3"=w993, "error in (no error)"=w989, "reference 4"=w992, "reference 5"=w991) -> ("camout"=w987:i32[], "error out"=w990:errorcluster)  [unwired: 6 in]
              }
            }
            n533 = Unbundle By Name(w860) -> ("status"=w972:bool)
            n534 = Not(x=w972) -> (.not. x?=w971:bool)
            n535 = case shown="True" w971 {
              tunnel: [w1061 w1064] -> w859
              tunnel: w860 -> [w1062 w1073]
              tunnel: w857 -> [w1063 w1084]
              tunnel: [w1063 w1083] -> w970
              tunnel: w892 -> [w1056 w1072]
              tunnel: w967 -> [_ w1080]
              tunnel: w935 -> [_ w1079]
              tunnel: [w1060 w1078] -> w966
              tunnel: [w1060 w1077] -> w965
              tunnel: w960 -> [w1059 w1076]
              tunnel: [w1059 w1075] -> w959
              tunnel: [i64 0 ("Num Records Total") w1074] -> w958
              tunnel: [dbl[] [] w1069] -> w927
              tunnel: [0 w1068] -> w926
              frame False {
                w1060 = FALSE ("Stop Measurement")
                n536 = call "HH_Stop.vi"("Device Index"=w1056, "error in (no error)"=w1062) -> ("error out"=w1061:errorcluster)  [unwired: 12 in, 1 out]
              }
              frame True {
                # "Overflow Interv. Time (s)"
                # "No Error"
                n537 = Initialize Array(0, 5) -> (w1067:i32[])
                n538 = while {
                  tunnel: w1072 -> [w1093]
                  tunnel: w1080 -> [w1117]
                  tunnel: w1079 -> [w1116]
                  shift-right: [w1094] -> w1082
                  shift-left: w1073 -> [w1118]
                  shift-right: [w1115] -> w1083
                  shift-left: w1084 -> [w1115]
                  shift-right: [FALSE ("Reset")] -> _
                  shift-left: TRUE ("Reset") -> [w1111]
                  tunnel: [w1108] -> w1078
                  tunnel: [w1100] -> w1077
                  tunnel: w1076 -> [w1104]
                  tunnel: [w1103] -> w1075
                  tunnel: [w1102] -> w1074
                  tunnel: [w1101] -> w1068
                  shift-right: [w1088] -> w1070
                  shift-left: w1067 -> [w1087]
                  tunnel: [w1085] -> w1071
                  i -> [w1086]
                  stop <- w1114 stop-if-true
                  n539 = call "HH_FIFORead.vi"("Device Index"=w1093, "Buffer In"=w1117, "Count"=w1116, "error in (no error)"=w1118) -> ("OK"=w1109:bool, "Buffer Out"=w1105:u32[], "Data Count"=w1106:i32, "FiFo Overrun"=w1108:bool, "error out"=w1107:errorcluster)  [unwired: 7 in]
                  n540 = Wait (ms)(milliseconds to wait=u32 10) -> ()  [unwired: 1 out]
                  n541 = local write "Buffer Overrun"(w1108) -> ()
                  n542 = Unbundle(w1107) -> ("status"=w1113:bool)  [unwired: 2 out]
                  n543 = call "HT3_Write.vi"("error in"=w1107, "Data Count"=w1106, "Data in"=w1105, "refnum in"=w1104) -> ("error out"=w1095:errorcluster, "refnum out"=w1103:refnum<file>)  [unwired: 6 in]
                  n544 = call "HH_TraceAndHisto.vi"("Data In"=w1105, "Reset"=w1111, "Data Count"=w1106) -> ("Histograms"=w1097:i32[][], "Total Oveflow Count"=w1101:u64, "Num Records Total"=w1102:i64, "Traces"=w1096:i32[][])  [unwired: 8 in, 1 out]
                  n545 = local read "Stop Measurement"() -> (w1099:bool)
                  n546 = local read "Global Stop"() -> (w1098:bool)
                  n547 = local write "Trace"(w1096) -> ()
                  n548 = call "GetCountRates.vi"("error in (no error)"=w1095, "DeviceIndex"=w1093) -> ("error out"=w1094:errorcluster, "CntRates"=w1089:dbl[], "SyncRate"=w1090:i32)  [unwired: 1 in]
                  n549 = local write "Histogram"(w1097) -> ()
                  n550 = Compound Arithmetic op=OR(invert w1109, w1113, w1098, w1099) -> (w1114:bool)
                  n551 = Insert Into Array(array=w1089, index=0, new element=w1090) -> (w1091:dbl[])
                  n552 = Or(x=w1099, y=w1098) -> (x .or. y?=w1100:bool)
                  n553 = Add(x=w1087, y=w1091) -> (x+y=w1088:dbl[])
                  n554 = Increment(x=w1086) -> (x+1=w1085:i32)
                }
                n555 = Divide(x=w1070, y=w1071) -> (x/y=w1069:dbl[])
                n556 = call "HH_Stop.vi"("Device Index"=w1072, "error in (no error)"=w1082) -> ("error out"=w1064:errorcluster)  [unwired: 12 in, 1 out]
              }
            }
            n557 = Reshape Array(w849, w848, w847) -> (w841:i32[][])
            n558 = property on="Point" class="IntGraph (strict)"(error in=w840, "Value"=w841) -> (error out=w839:errorcluster)  [unwired: 1 in, 1 out]
            n559 = Merge Errors(w859, w839) -> (w858:errorcluster)
            n560 = call "AOTF-Trigger_1.vi"("Channel"=w921, "Pulse length"=w912, "Sync trigger ratio"=5, "error in (no error)"=w856, "Triggered"=FALSE) -> ("error out"=w930:errorcluster)  [unwired: 2 in]
            n561 = call "MOV.vi"("System no."=w887, "Axes to move"=w881, "Position values"=w880, "error in"=w905) -> ("error out"=w904:errorcluster)  [unwired: 15 in]
          }
          frame "Save Color Image" {
            n562 = local read "Active pt3"() -> (w1126:path)
            n563 = call "MTS_GetFileFromWS.vi"(".pt3 File Name"=w1126) -> ("File Header"=w1125:T39)  [unwired: 9 in, 1 out]
            n564 = Unbundle By Name(w1125) -> ("Measurement Type"=w1124:T40, "Pixels"=w1121:i32[])
            n565 = control-ref of="WS File Tree"() -> (w1127:refnum<vi>)
            n566 = Equal?(x=T29."Image File" ("Measurement Type"), y=w1124) -> (x = y?=w1122:bool)
            n567 = case shown="True" w1122 {
              tunnel: w1130 -> [w1131 w1154]
              tunnel: w1126 -> [_ w1153]
              tunnel: w1126 -> [_ _]
              tunnel: [w1131 w1133] -> w1119
              tunnel: w1127 -> [_ _]
              tunnel: w1121 -> [_ w1138]
              frame False {
              }
              frame True {
                # "Image Intensity Array"
                # "Image Intensity Array"
                n568 = call "HT3_Open.vi"("error in"=w1154, "File Path"=w1153) -> ("error out"=w1146:errorcluster, "Header"=w1150:T41, "refnum out"=w1152:refnum<file>)  [unwired: 3 in, 4 out]
                n569 = Unbundle By Name(w1150) -> ()  [unwired: 15 out]
                n570 = Index Array(array=w1138, index #2=1 ("index")) -> (element #1=w1135:i32, element #2=w1136:i32)  [unwired: 1 in]
                n571 = Initialize Array(0 ("element"), w1135, w1136) -> (w1148:i32[][])
                n572 = Initialize Array(0 ("element"), 4 ("dimension size"), w1135, w1136) -> (w1141:i32[][][])
                n573 = while {
                  tunnel: w1152 -> [w1179]
                  shift-right: [FALSE ("Start From Top")] -> _
                  shift-left: TRUE ("Start From Top") -> [w1173]
                  shift-right: [w1172] -> w1145
                  shift-left: w1146 -> [w1170]
                  tunnel: [w1171] -> w1144
                  tunnel: w1148 -> [w1169]
                  tunnel: [w1168] -> w1147
                  tunnel: [w1169] -> _
                  stop <- w1176 stop-if-true
                  n574 = call "HT3_Read.vi"("Start From Top"=w1173, "error in"=w1170, "Data count"=10000, "refnum in"=w1179) -> ("error out"=w1172:errorcluster, "Data out"=w1175:u32[], "refnum out"=w1171:refnum<file>, "EOF?"=w1176:bool)  [unwired: 4 in]
                  n575 = Array Size(array=w1175) -> (size(s)=w1174:i32)
                  n576 = call "HH_FileToImage_1.vi"("Data In"=w1175, "Reset"=w1173, "Data Count"=w1174) -> ("Histograms"=w1168:i32[][])  [unwired: 7 in, 5 out]
                }
                n577 = call "MTS_SelectTCSPCBinning.vi"("Histograms in"=w1147) -> ("TCSPC Binning"=w1140:i32[][])  [unwired: 1 in, 9 out]
                n578 = while {
                  tunnel: w1144 -> [w1167]
                  shift-right: [FALSE ("Start From Top")] -> _
                  shift-left: TRUE ("Start From Top") -> [w1161]
                  shift-right: [w1160] -> w1132
                  shift-left: w1145 -> [w1156]
                  tunnel: [w1159] -> w1134
                  tunnel: w1141 -> [w1158]
                  tunnel: [w1157] -> _
                  tunnel: w1140 -> [w1155]
                  stop <- w1164 stop-if-true
                  n579 = call "HT3_Read.vi"("Start From Top"=w1161, "error in"=w1156, "Data count"=10000, "refnum in"=w1167) -> ("error out"=w1160:errorcluster, "Data out"=w1163:u32[], "refnum out"=w1159:refnum<file>, "EOF?"=w1164:bool)  [unwired: 4 out]
                  n580 = Array Size(array=w1163) -> (size(s)=w1162:i32)
                  n581 = call "HH_ToColorImage.vi"("Data In"=w1163, "Reset"=w1161, "Image Array In"=w1158, "Data Count"=w1162, "TCSPC Binning"=w1155) -> ("Image Array Out"=w1157:i32[][][])  [unwired: 2 in, 8 out]
                }
                n582 = Close File(refnum=w1134, error in=w1132) -> (error out=w1133:errorcluster)  [unwired: 1 out]
              }
            }
          }
          frame "Find Single Mol." {
            # "dirty trick"
            n583 = local read "Active pt3"() -> (w1206:path)
            n584 = call "MTS_GetFileFromWS.vi"(".pt3 File Name"=w1206) -> ("File Header"=w1205:T39)  [unwired: 9 in, 1 out]
            n585 = Unbundle By Name(w1205) -> ("Measurement Type"=w1204:T40, "Pixels"=w1192:i32[], "Upper Left"=w1201:T42, "Scan Axis"=w1200:enum32{"x-y", "x-z", "y-z"})
            n586 = local read "Picture size 2"() -> (w1187:dbl)
            n587 = local read "Picture size"() -> (w1190:dbl)
            n588 = local read "Resolution"() -> (w1188:dbl)
            n589 = local read "X-Position"() -> (w1181:dbl)
            n590 = local read "Y-Position"() -> (w1180:dbl)
            n591 = Divide(x=w1190, y=w1188) -> (x/y=w1189:dbl)
            n592 = Divide(x=w1187, y=w1188) -> (x/y=w1186:dbl)
            n593 = Equal?(x=T29."Image File" ("Measurement Type"), y=w1204) -> (x = y?=w1202:bool)
            n594 = call "MTS_ScannerXYZToImageXY.vi"("Axis"=w1200, "Scanner XYZ"=w1201) -> ("Image Y"=w1183:dbl, "Image X"=w1185:dbl)
            n595 = case shown="True" TRUE {
              tunnel: [w1209 w1212] -> w1191
              tunnel: w1192 -> [w1209 _]
              tunnel: w1189 -> [_ w1216]
              tunnel: w1186 -> [_ w1215]
              tunnel: [w1208 w1211] -> w1184
              tunnel: w1185 -> [w1208 _]
              tunnel: [w1207 w1210] -> w1182
              tunnel: w1183 -> [w1207 _]
              tunnel: w1181 -> [_ w1211]
              tunnel: w1180 -> [_ w1210]
              frame False {
              }
              frame True {
                n596 = To Long Integer(number=w1216) -> (32bit integer=w1214:i32)
                n597 = To Long Integer(number=w1215) -> (32bit integer=w1213:i32)
                n598 = Build Array(w1214, w1213) -> (w1212:i32[])
              }
            }
            n599 = Build Array(w1190, w1187) -> (w1196:dbl[])
            n600 = case shown="True" w1202 {
              tunnel: w1199 -> [w1217 w1293]
              tunnel: w1206 -> [_ _]
              tunnel: w1206 -> [_ _]
              tunnel: [w1217 w1298] -> w1197
              tunnel: w1191 -> [_ w1315]
              tunnel: w1196 -> [_ w1297]
              tunnel: w1184 -> [_ w1307]
              tunnel: w1182 -> [_ w1308]
              frame False {
              }
              frame True {
                w1267 = T11 1 items=["Center of Mass X", "Center of Mass Y", "First Pixel X", "First Pixel Y", "Bounding Rect Left", "Bounding Rect Top", "Bounding Rect Right", "Bounding Rect Bottom", "Max Feret Diameter Start X", "Max Feret Diameter Start Y", "Max Feret Diameter End X", "Max Feret Diameter End Y", "Max Horiz. Segment Length Left", "Max Horiz. Segment Length Right", "Max Horiz. Segment Length Row", "-", "Bounding Rect Width", "Bounding Rect Height", "Bounding Rect Diagonal", "Perimeter", "Convex Hull Perimeter", "Holes' Perimeter", "Max Feret Diameter", "Equivalent Ellipse Major Axis", "Equivalent Ellipse Minor Axis", "Equivalent Ellipse Minor Axis (Feret)", "Equivalent Rect Long Side", "Equivalent Rect Short Side", "Equivalent Rect Diagonal", "Equivalent Rect Short Side (Feret)", "Average Horiz. Segment Length", "Average Vert. Segment Length", "Hydraulic Radius", "Waddel Disk Diameter", "-", "Area", "Holes' Area", "Particle & Holes' Area", "Convex Hull Area", "Image Area", "-", "Number of Holes", "Number of Horiz. Segments", "Number of Vert. Segments", "-", "Orientation", "Max Feret Diameter Orientation", "-", "% Area/Image Area", "% Area/(Particle & Holes' Area)", "Ratio of Equivalent Ellipse Axes", "Ratio of Equivalent Rect Sides", "-", "Elongation Factor", "Compactness Factor", "Heywood Circularity Factor", "Type Factor", "-", "Sum X", "Sum Y", "Sum XX", "Sum XY", "Sum YY", "Sum XXX", "Sum XXY", "Sum XYY", "Sum YYY", "-", "Moment of Inertia XX", "Moment of Inertia XY", "Moment of Inertia YY", "Moment of Inertia XXX", "Moment of Inertia XXY", "Moment of Inertia XYY", "Moment of Inertia YYY", "Norm. Moment of Inertia XX", "Norm. Moment of Inertia XY", "Norm. Moment of Inertia YY", "Norm. Moment of Inertia XXX", "Norm. Moment of Inertia XXY", "Norm. Moment of Inertia XYY", "Norm. Moment of Inertia YYY", "Hu Moment 1", "Hu Moment 2", "Hu Moment 3", "Hu Moment 4", "Hu Moment 5", "Hu Moment 6", "Hu Moment 7"] ("Measurement Parameter")
                w1248 = TRUE ("Measurement Type")
                w1272 = T11 0 items=["Center of Mass X", "Center of Mass Y", "First Pixel X", "First Pixel Y", "Bounding Rect Left", "Bounding Rect Top", "Bounding Rect Right", "Bounding Rect Bottom", "Max Feret Diameter Start X", "Max Feret Diameter Start Y", "Max Feret Diameter End X", "Max Feret Diameter End Y", "Max Horiz. Segment Length Left", "Max Horiz. Segment Length Right", "Max Horiz. Segment Length Row", "-", "Bounding Rect Width", "Bounding Rect Height", "Bounding Rect Diagonal", "Perimeter", "Convex Hull Perimeter", "Holes' Perimeter", "Max Feret Diameter", "Equivalent Ellipse Major Axis", "Equivalent Ellipse Minor Axis", "Equivalent Ellipse Minor Axis (Feret)", "Equivalent Rect Long Side", "Equivalent Rect Short Side", "Equivalent Rect Diagonal", "Equivalent Rect Short Side (Feret)", "Average Horiz. Segment Length", "Average Vert. Segment Length", "Hydraulic Radius", "Waddel Disk Diameter", "-", "Area", "Holes' Area", "Particle & Holes' Area", "Convex Hull Area", "Image Area", "-", "Number of Holes", "Number of Horiz. Segments", "Number of Vert. Segments", "-", "Orientation", "Max Feret Diameter Orientation", "-", "% Area/Image Area", "% Area/(Particle & Holes' Area)", "Ratio of Equivalent Ellipse Axes", "Ratio of Equivalent Rect Sides", "-", "Elongation Factor", "Compactness Factor", "Heywood Circularity Factor", "Type Factor", "-", "Sum X", "Sum Y", "Sum XX", "Sum XY", "Sum YY", "Sum XXX", "Sum XXY", "Sum XYY", "Sum YYY", "-", "Moment of Inertia XX", "Moment of Inertia XY", "Moment of Inertia YY", "Moment of Inertia XXX", "Moment of Inertia XXY", "Moment of Inertia XYY", "Moment of Inertia YYY", "Norm. Moment of Inertia XX", "Norm. Moment of Inertia XY", "Norm. Moment of Inertia YY", "Norm. Moment of Inertia XXX", "Norm. Moment of Inertia XXY", "Norm. Moment of Inertia XYY", "Norm. Moment of Inertia YYY", "Hu Moment 1", "Hu Moment 2", "Hu Moment 3", "Hu Moment 4", "Hu Moment 5", "Hu Moment 6", "Hu Moment 7"] ("Measurement Parameter")
                w1287 = T43 4 items=["Grayscale (U8)", "Grayscale (I16)", "Grayscale (SGL)", "Complex (CSG)", "RGB (U32)", "HSL (U32)", "RGB (U64)", "Grayscale (U16)"] ("Image Type")
                w1295 = T43 4 items=["Grayscale (U8)", "Grayscale (I16)", "Grayscale (SGL)", "Complex (CSG)", "RGB (U32)", "HSL (U32)", "RGB (U64)", "Grayscale (U16)"] ("Image Type")
                w1314 = 1 ("index")
                # "Pixel Size [um]"
                n601 = Index Array(array=w1297, index #2=w1314) -> (element #1=w1313:dbl, element #2=w1310:dbl)  [unwired: 1 in]
                n602 = Index Array(array=w1315, index #2=w1314) -> (element #1=w1312:i32, element #2=w1311:i32)  [unwired: 1 in]
                n603 = Divide(x=w1313, y=w1312) -> (x/y=w1219:dbl)
                n604 = Divide(x=w1310, y=w1311) -> (x/y=w1309:dbl)
                n605 = Reciprocal(x=w1219) -> (1/x=w1224:dbl)
                n606 = Multiply(x=w1224, y="Focuswidth") -> (x*y=w1223:dbl)
                n607 = Random Number (0-1)() -> (number: 0 to 1=w1292:dbl)
                n608 = Number To Decimal String(number=w1292) -> (decimal integer string=w1291:string)  [unwired: 1 in]
                n609 = Concatenate Strings(w1291, "IMAQ CreatePatternimg" ("Image Name")) -> (w1289:string)
                n610 = call "IMAQ Create"("Image Name"=w1289, "Image Type"=w1295, "error in (no error)"=w1293) -> ("New Image"=w1294:T5, "error out"=w1282:errorcluster)  [unwired: 2 in]
                n611 = local read "Image"() -> (w1226:i32[][])
                n612 = call "MTS_IntensityArrayToImage.vi"(0:"Image"=w1294, 1:"Image"=w1226, "error in (no error)"=w1282, "Log Scale"=FALSE) -> ("Image Out"=w1247:T5, "error out"=w1239:errorcluster)  [unwired: 10 in]
                n613 = Random Number (0-1)() -> (number: 0 to 1=w1286:dbl)
                n614 = Array To Cluster(array=T32 [] ("MesaurementSelection")) -> (cluster=w1275:T44)
                n615 = Number To Decimal String(number=w1286) -> (decimal integer string=w1285:string)  [unwired: 1 in]
                n616 = Unbundle By Name(w1275) -> ("MesaurementSelection[0]"=w1273:T45, "MesaurementSelection[1]"=w1268:T45, "MesaurementSelection[2]"=w1263:T45, "MesaurementSelection[3]"=w1254:T45)
                n617 = Concatenate Strings(w1285, "IMAQ CreatePatternimg2" ("Image Name")) -> (w1283:string)
                n618 = call "IMAQ Create"("Image Name"=w1283, "Image Type"=w1287, "error in (no error)"=w1239) -> ("New Image"=w1281:T5, "error out"=w1238:errorcluster)  [unwired: 2 in]
                n619 = Bundle By Name(cluster=w1273, "Measurement Parameter"=w1272, "Range Lower Value"="X Start 2", "Range Upper Value"="X End 2", "Range"="Exclude / Include X", "Measurement Type"=w1248) -> (w1262:T45)
                n620 = Bundle By Name(cluster=w1268, "Measurement Parameter"=w1267, "Range Lower Value"="Y Start 2", "Range Upper Value"="Y End 2", "Range"="Exclude / Include Y", "Measurement Type"=w1248) -> (w1261:T45)
                n621 = Bundle By Name(cluster=w1263, "Measurement Parameter"="Measurement Parameter 1", "Range Lower Value"="Range Lower Value Par 1", "Range Upper Value"="Range Upper Value  Par 1", "Range"="Ex/In Par 1", "Measurement Type"=w1248) -> (w1260:T45)
                n622 = Bundle By Name(cluster=w1254, "Measurement Parameter"="Measurement Parameter 2", "Range Lower Value"="Range Lower Value Par 2", "Range Upper Value"="Range Upper Value Par 2", "Range"="Ex/In Par 2", "Measurement Type"=w1248) -> (w1253:T45)
                n623 = Build Array(w1262, w1261, w1260, w1253) -> (w1259:T32)
                n624 = call "MTS_IntensityArrayToImage.vi"(0:"Image"=w1281, 1:"Image"=w1226, "error in (no error)"=w1238, "Log Scale"=TRUE) -> ("Image Out"=w1232:T5, "error out"=w1237:errorcluster)  [unwired: 10 in]
                n625 = case shown="0, Default" "Detection Modus" {
                  tunnel: "Remove Outliers" -> [_ w1349]
                  tunnel: [w1326 w1340] -> w1288
                  tunnel: w1237 -> [w1331 w1348]
                  tunnel: [w1324 w1338] -> w1279
                  tunnel: "Filter" -> [_ w1347]
                  tunnel: w1259 -> [_ w1346]
                  tunnel: w1247 -> [_ w1341]
                  tunnel: path "C:/Users/Core-FCS/Desktop/Documents/AbelFCS/ParticleFinder/SingleMoleculePatternFinder/Patterns/azimutalGolden.png" ("Template File Path (GeometricMatching)") -> [_ _]
                  tunnel: "Settings (GeometricMatching)" -> [_ _]
                  tunnel: IMAQ_Rounding_Mode."Optimize" ("Rounding Mode Gaussian") -> [_ w1345]
                  tunnel: IMAQ_Rounding_Mode."Optimize" ("Rounding Mode Convolution") -> [_ w1344]
                  tunnel: "Square/Hexa" -> [_ w1343]
                  tunnel: "Connectivity 4/8" -> [_ w1342]
                  tunnel: w1232 -> [w1328 w1336]
                  tunnel: [w1328 w1333] -> w1236
                  tunnel: [w1330 w1334] -> w1234
                  tunnel: "Manual" -> [_ w1332]
                  tunnel: w1226 -> [w1322 _]
                  tunnel: "Mode" -> [w1321 _]
                  tunnel: w1223 -> [w1320 _]
                  tunnel: [w1319 _] -> w1221
                  tunnel: "NA" -> [w1318 _]
                  tunnel: w1219 -> [w1317 _]
                  tunnel: "TSH" -> [w1316 _]
                  frame 0, Default {
                    n626 = To Double Precision Float(number=w1322) -> (double precision float=w1323:dbl[][])
                    n627 = script code="addpath(path);\nswitch (mode)\ncase 0\nmaskGauss = GenGauss2D(focus);\n[err,bim,cim,sim,yc,xc,bc,cc,sc,len,imm]=FindPatternCP(image,maskGauss,[],[],[],tsh);\npattern=maskGauss;\ncase 1\nmaskRad=Radialpattern_gen('radial', Pixel,NA);\n[err,bim,cim,sim,yc,xc,bc,cc,sc,len,imm]=FindPatternCP(image,maskRad,[],[],[],tsh);\npattern=maskRad(:,:,15);\ncase 2\nmaskAzi=Radialpattern_gen('azimuthal', Pixel,NA);\n[err,bim,cim,sim,yc,xc,bc,cc,sc,len,imm]=FindPatternCP(image,maskAzi,[],[],[],tsh);\npattern=maskAzi(:,:,15);\nend\nxc=xc-1;\nyc=yc-1;"("??"=w1331, "path"="C:\\Users\\Core-FCS\\Desktop\\Documents\\CoreSetupNew\\MatlabLibAbelFCS", "image"=w1323, "mode"=w1321, "focus"=w1320, "NA"=w1318, "Pixel"=w1317, "tsh"=w1316) -> ("??"=w1330:errorcluster, "pattern"=w1319:dbl[][], "xc"=w1327:dbl[], "yc"=w1325:dbl[])
                    n628 = Build Array(w1327, w1325) -> (w1326:dbl[][])
                    n629 = Array Size(array=w1325) -> (size(s)=w1324:i32)
                  }
                  frame 1 {
                    n630 = call "SingleMoleFinderEasy.vi"("Image Src"=w1341, "Number of Erosion"=w1349, "HolesBorder"=w1347, "Selection Values"=w1346, "Rounding Mode Gaussian"=w1345, "error in"=w1348, "Rounding Mode Convolution"=w1344, "Square/Hexa (Square)"=w1343, "Connectivity 4/8 (8)"=w1342) -> ("Number of Particles"=w1337:i32, "Particle Measurements (Pixels)"=w1339:dbl[][], "error out"=w1335:errorcluster)  [unwired: 15 in, 1 out]
                    n631 = case shown="True" w1332 {
                      tunnel: w1335 -> [w1353 w1361]
                      tunnel: [w1353 w1360] -> w1334
                      tunnel: [w1350 w1359] -> w1333
                      tunnel: [w1351 w1358] -> w1340
                      tunnel: w1339 -> [w1351 w1355]
                      tunnel: [w1352 w1357] -> w1338
                      tunnel: w1337 -> [w1352 w1356]
                      tunnel: w1336 -> [w1350 w1354]
                      frame False {
                      }
                      frame True {
                        n632 = while {
                          tunnel: w1361 -> [w1376]
                          tunnel: [w1375] -> w1360
                          tunnel: w1354 -> [w1374]
                          tunnel: [w1373] -> w1359
                          shift-right: [w1366] -> w1358
                          shift-left: w1355 -> [w1365]
                          tunnel: [w1364] -> w1357
                          tunnel: w1356 -> [w1363]
                          i -> [w1370]
                          stop <- w1372 stop-if-true
                          n633 = call "IMAQ Select Point"("Window Number (0...15)"=1, "error in (no error)"=w1376, "Image In"=w1374) -> ("error out"=w1375:errorcluster, "Cancelled"=w1372:bool, "Point"=w1371:T46, "Image Out (duplicate)"=w1373:T5)  [unwired: 5 in]
                          n634 = Unbundle(w1371) -> ("X"=w1369:sgl, "Y"=w1368:sgl)
                          n635 = Build Array(w1369, w1368) -> (w1367:sgl[])
                          n636 = Add(x=w1363, y=w1370) -> (x+y=w1364:i32)
                          n637 = Insert Into Array(array=w1365, index (row)=w1364, new element=w1367) -> (w1366:dbl[][])  [unwired: 1 in]
                        }
                      }
                    }
                  }
                }
                "Number of Particles" <- w1279
                "Image 2" <- w1221
                n638 = Index Array(array=w1288, index (col) #1=0 ("index (row)"), index (col) #2=1 ("index (col)")) -> (element #1=w1231:dbl[], element #2=w1229:dbl[])  [unwired: 2 in]
                n639 = Multiply(x=w1219, y=w1231) -> (x*y=w1306:dbl[])
                n640 = Multiply(x=w1229, y=w1309) -> (x*y=w1305:dbl[])
                n641 = To Word Integer(number=w1231) -> (16bit integer=w1230:i16[])
                n642 = To Word Integer(number=w1229) -> (16bit integer=w1228:i16[])
                n643 = Add(x=w1307, y=w1306) -> (x+y=w1301:dbl[])
                n644 = Add(x=w1305, y=w1308) -> (x+y=w1300:dbl[])
                n645 = for {
                  N: w1279 -> [_]
                  shift-right: [w1383] -> w1235
                  shift-left: w1236 -> [w1384]
                  tunnel: w1230 -> [w1382] mode=indexing
                  tunnel: w1228 -> [w1381] mode=indexing
                  shift-right: [w1385] -> w1233
                  shift-left: w1234 -> [w1386]
                  tunnel: u32 16738560 -> [w1380]
                  tunnel: 3.0 ("x") -> [w1379]
                  n646 = call "MTS_DrawCrossIMAQIamge.vi"("Image"=w1384, "Size"=w1379, "Color"=w1380, "X"=w1382, "Y"=w1381, "error in (no error)"=w1386) -> ("Image Out"=w1383:T5, "error out"=w1385:errorcluster)  [unwired: 8 in]
                }
                "AM image" <- w1235
                n647 = Build Array(w1301, w1300, w1230, w1228) -> (→"Pattern":dbl[][])
                n648 = global write "patternImg.vi" "New Image"(w1235) -> ()
                n649 = flat-sequence {
                  tunnel: w1233 -> [w1378]
                  tunnel: [w1378] -> w1298
                  frame #0 {
                    n650 = local write "Tab Control"(T4."AutoMesaurement" ("Tab Control")) -> ()
                  }
                }
              }
            }
          }
          frame "Auto Measurement Control" {
            # "Init"
            n651 = local read "Pattern"() -> (w1397:dbl[][])
            n652 = Index Array(array=w1397, index (row) #1=2 ("index (row)"), index (row) #2=3 ("index (col)")) -> (element #1=w1394:dbl[], element #2=→"subarray":dbl[])  [unwired: 2 in]
            n653 = local read "NxtAutMesPoint"() -> (w1405:i32)
            n654 = Array Size(array=w1394) -> (size(s)=w1393:i32)
            n655 = Less Than 0?(x=w1405) -> (x < 0?=w1408:bool)
            n656 = case shown="False" w1408 {
              tunnel: w1402 -> [w1429 w1433]
              tunnel: [w1429 w1432] -> w1406
              tunnel: [w1428 w1430] -> w1404
              tunnel: w1393 -> [_ w1430]
              frame False {
                n657 = local read "Auto Measure Points"() -> (w1428:i32)
              }
              frame True {
                n658 = Number To Decimal String(number=w1430) -> (decimal integer string=w1435:string)  [unwired: 1 in]
                n659 = Concatenate Strings("Point 1 / " ("Caption.Text"), w1435) -> (w1434:string)
                n660 = property on="Auto Meas Progress" class="Slide (strict)"(error in=w1433, "Scale.Minimum"=0.0 ("Scale.Range:Minimum"), "Scale.Maximum"=w1430, "Value"=1 ("Auto Meas Progress"), "Caption.Text"=w1434) -> (error out=w1432:errorcluster)  [unwired: 1 in, 1 out]
                "Auto Measure Points" <- w1430
              }
            }
            n661 = Increment(x=w1405) -> (x+1=w1388:i32)
            "NxtAutMesPoint" <- w1388
            n662 = Greater Or Equal?(x=w1388, y=w1404) -> (x >= y?=w1407:bool)
            n663 = Increment(x=w1388) -> (x+1=w1403:i32)
            n664 = Index Array(array=w1397, index (row) #1=2 ("index (row)"), index (col) #1=w1388, index (row) #2=3 ("index (col)"), index (col) #2=w1388) -> (element #1=w1396:dbl, element #2=w1395:dbl)
            n665 = case shown="False" w1407 {
              tunnel: w1406 -> [w1419 w1427]
              tunnel: [w1425 w1427] -> w1400
              tunnel: [T14."Auto Point" ("Do Measurement") T14."No Measurement" ("Do Measurement")] -> w1399
              tunnel: w1403 -> [w1420 _]
              tunnel: w1396 -> [w1417 _]
              tunnel: w1395 -> [w1416 _]
              tunnel: w1404 -> [w1413 _]
              frame False {
                # "Prpare For Next Point"
                # "1 loc max  2 undef 0 saddle -1 local min"
                n666 = global read "patternImg.vi" "New Image"() -> (w1409:T5)
                n667 = Number To Decimal String(number=w1420) -> (decimal integer string=w1422:string)  [unwired: 1 in]
                n668 = Number To Decimal String(number=w1413) -> (decimal integer string=w1414:string)  [unwired: 1 in]
                n669 = Concatenate Strings("Point " ("Caption.Text"), w1422, " / " ("Caption.Text"), w1414) -> (w1421:string)
                n670 = call "MTS_DrawCrossIMAQIamge.vi"("Image"=w1409, "Size"=3.0 ("x"), "Color"=u32 6618880, "X"=w1417, "Y"=w1416, "error in (no error)"=w1419) -> ("Image Out"=w1410:T5, "error out"=w1418:errorcluster)  [unwired: 8 in]
                n671 = local write "AM image"(w1410) -> ()
                n672 = property on="Auto Meas Progress" class="Slide (strict)"(error in=w1418, "Value"=w1420, "Caption.Text"=w1421) -> (error out=w1425:errorcluster)  [unwired: 1 in, 1 out]
              }
              frame True {
                # "No More Points"
              }
            }
          }
        }
        n673 = local write "Buffer Overrun"(w574) -> ()
      }
      frame Error {
      }
    }
    n674 = Unbundle(w559) -> ("status"=w558:bool)  [unwired: 2 out]
    n675 = flat-sequence {
      tunnel: w562 -> [w1453]
      tunnel: [w1453] -> w561
      tunnel: w557 -> [w1450]
      frame #0 {
        n676 = local write "Task"(w1450) -> ()
        n677 = Equal?(x=w1450, y=T25."No Measurement" ("Do Measurement")) -> (x = y?=w1451:bool)
        n678 = Not(x=w1451) -> (.not. x?=w1452:bool)
        n679 = local write "Running"(w1452) -> ()
      }
    }
    n680 = local read "Global Stop"() -> (w565:bool)
    n681 = Compound Arithmetic op=OR(w558, w563, w565) -> (w564:bool)
  }
  n682 = while {
    tunnel: w6 -> [w1454]
    tunnel: [w1455] -> _
    stop <- w1458 stop-if-true
    n683 = property on="3dAbelFcs" class="Bool (strict)"(error in=w1454) -> (error out=w1456:errorcluster, "Value"=w1457:bool)  [unwired: 1 in, 1 out]
    n684 = local read "Global Stop"() -> (w1458:bool)
    n685 = case shown="False" w1457 {
      tunnel: w1456 -> [_ w1467]
      tunnel: [_ w1473] -> w1455
      frame False {
      }
      frame True {
        n686 = local read "Z Stepsize"() -> (w1470:dbl)
        n687 = local read "Y Stepsize"() -> (w1471:dbl)
        n688 = local read "X Stepsize"() -> (w1472:dbl)
        n689 = local read "Z Steps"() -> (w1469:dbl)
        n690 = call "SetShutter.vi"("type"=Shutter_type_typedef."TTL High", "mode"=Shutter_mode_typedef."Open", "error in (no error)"=w1467) -> ("error out"=w1459:errorcluster)  [unwired: 11 in, 1 out]
        n691 = for {
          N: w1469 -> [_]
          tunnel: w1459 -> [w1483]
          tunnel: w1470 -> [w1488]
          tunnel: w1471 -> [w1487]
          tunnel: w1472 -> [w1486]
          tunnel: [w1482] -> w1468
          tunnel: w1469 -> [w1481]
          i -> [w1485]
          n692 = local read "Z Start"() -> (w1475:dbl)
          n693 = local write "Z-Position"(w1475) -> ()
          n694 = Multiply(x=w1488, y=w1485) -> (x*y=w1479:dbl)
          n695 = Subtract(x=200, y=w1475) -> (x-y=w1476:dbl)
          n696 = local read "Y Steps"() -> (w1480:dbl)
          n697 = Add(x=w1476, y=w1479) -> (x+y=w1477:dbl)
          n698 = Number To Decimal String(number=w1485) -> (decimal integer string=w1484:string)  [unwired: 1 in]
          n699 = for {
            N: w1480 -> [_]
            tunnel: w1487 -> [w1526]
            tunnel: w1486 -> [w1525]
            tunnel: w1483 -> [w1522]
            tunnel: w1484 -> [w1524]
            tunnel: [w1496] -> w1482
            tunnel: w1475 -> [w1493]
            tunnel: w1481 -> [w1517]
            tunnel: w1480 -> [w1516]
            tunnel: w1477 -> [w1514]
            i -> [w1498]
            w1494 = "_" ("string")
            n700 = local read "X Steps"() -> (w1515:dbl)
            n701 = Number To Decimal String(number=w1498) -> (decimal integer string=w1523:string)  [unwired: 1 in]
            n702 = for {
              N: w1515 -> [_]
              tunnel: w1522 -> [w1541]
              tunnel: w1525 -> [w1546]
              tunnel: [w1542] -> w1520
              tunnel: w1524 -> [w1544]
              tunnel: w1523 -> [w1543]
              shift-right: [w1540] -> w1519
              shift-left: _ -> [w1539]
              tunnel: [w1538] -> w1518
              tunnel: [w1536] -> w1513
              tunnel: [w1537] -> w1512
              i -> [w1545]
              n703 = control-ref of="Stop Measurement"() -> (w1532:refnum<vi>)
              n704 = control-ref of="Point Measurement"() -> (w1527:refnum<vi>)
              n705 = control-ref of="Running"() -> (w1535:refnum<vi>)
              n706 = control-ref of="FCS Point Measurement"() -> (w1530:refnum<vi>)
              n707 = control-ref of="concatenated string"() -> (w1528:refnum<vi>)
              n708 = control-ref of="Workspace"() -> (w1533:refnum<vi>)
              n709 = control-ref of="X-Position"() -> (w1531:refnum<vi>)
              n710 = control-ref of="X Start"() -> (w1529:refnum<vi>)
              n711 = control-ref of="Task"() -> (w1534:refnum<vi>)
              n712 = call "LifeTimeImagePoint.vi"("Boolean in"=w1535, "String"=w1543, "reference 6"=w1531, "String 2"=w1544, "reference 7"=w1530, "error in (no error)"=w1541, "reference 4"=w1532, "reference 3"=w1533, "reference 9"=w1529, "reference in"=w1534, "Numeric in"=w1545, "Str Refnum"=w1528, "X Stepsize"=w1546, "Array in"=w1539, "Point Measurement"=w1527) -> ("Array out"=w1540:i32[][], "CCD Chip Size"=w1537:i32, "X Start"=w1538:dbl, "Numeric out"=w1536:dbl, "error out"=w1542:errorcluster)  [unwired: 8 in]
            }
            n713 = property on="Workspace" class="Path"() -> ("Value"=w1495:path)  [unwired: 2 in, 2 out]
            n714 = Increment(x=w1498) -> (x+1=w1499:i32)
            n715 = Get Date/Time In Seconds() -> (seconds since 1Jan1904=w1504:timestamp)
            n716 = Strip Path(path=w1495) -> (stripped path=w1508:path)  [unwired: 1 out]
            n717 = Format Date/Time String(time format string (%c)="%d%m%y_%H%M", seconds (now)=w1504) -> (date/time string=w1502:string)  [unwired: 1 in]
            n718 = Path To String(path=w1508) -> (string=w1509:string)
            n719 = Number To Decimal String(number=w1499) -> (decimal integer string=w1505:string)  [unwired: 1 in]
            n720 = local read "Y Start"() -> (w1489:dbl)
            n721 = local write "Y-Position"(w1489) -> ()
            n722 = Concatenate Strings(w1509, "\\" ("string"), "AreaISM" ("string"), w1494, w1505, w1494, w1502, w1494, w1494) -> (w1510:string)
            n723 = Multiply(x=w1526, y=w1498) -> (x*y=w1521:dbl)
            n724 = Subtract(x=200, y=w1489) -> (x-y=w1490:dbl)
            n725 = Add(x=w1490, y=w1521) -> (x+y=w1491:dbl)
            n726 = String To Path(string=w1510) -> (path=w1501:path)
            n727 = Build Array(w1493, w1489, w1518, w1517, w1516, w1515, w1514, w1491, w1513, w1512) -> (w1511:dbl[])
            n728 = Path To String(path=w1501) -> (string=w1500:string)
            n729 = script code="results.ImagePlane=Data;\nresults.Info.Zstart=Meta(1);\nresults.Info.Ystart=Meta(2);\nresults.Info.Xstart=Meta(3);\nresults.Info.Zsteps=Meta(4);\nresults.Info.Ysteps=Meta(5);\nresults.Info.Xsteps=Meta(6);\nresults.Info.Zpos=Meta(7);\nresults.Info.Ypos=Meta(8);\nresults.Info.Xpos=Meta(9);\nresults.Info.CcdSize=Meta(13);\nsave(file,'results');\nclear results;"("??"=w1520, "Data"=w1519, "Meta"=w1511, "file"=w1500) -> ("??"=w1497:errorcluster)
            n730 = call "FreeInternalMemory.vi"("error in (no error)"=w1497) -> ("error out"=w1496:errorcluster)  [unwired: 1 in, 1 out]
          }
        }
        n731 = call "AbortAcquisition.vi"("error in (no error)"=w1468) -> ("error out"=w1465:errorcluster)  [unwired: 1 in, 1 out]
        n732 = call "SetShutter.vi"("type"=Shutter_type_typedef."TTL High", "mode"=Shutter_mode_typedef."Close", "error in (no error)"=w1465) -> ("error out"=w1461:errorcluster)  [unwired: 11 in, 1 out]
        n733 = call <vilib>:"Clear Errors.vi"("error in (no error)"=w1461) -> ("error out"=w1460:errorcluster)  [unwired: 6 in]
        n734 = property on="3dAbelFcs" class="Bool (strict)"(error in=w1460, "Value"=FALSE ("3dAbelFcs")) -> (error out=w1473:errorcluster)  [unwired: 1 in, 1 out]
      }
    }
  }
  n735 = call "PulseTrain.vi"("error in"=w6, "duty cycle"="duty cycle", "frequency"="frequency") -> ("error out"=w5:errorcluster, "task out"=w4:refnum<k21>)  [unwired: 7 in]
  n736 = while {
    tunnel: [w1547] -> w7
    tunnel: w5 -> [w1547]
    tunnel: w4 -> [w1548]
    tunnel: [w1548] -> w3
    stop <- w1550 stop-if-true
    n737 = Wait (ms)(milliseconds to wait=u32 100) -> ()  [unwired: 1 out]
    n738 = local read "Global Stop"() -> (w1550:bool)
  }
  n739 = call <vilib>:"DAQmx Clear Task.vi"("task in"=w3, "error in"=w7) -> ()  [unwired: 13 in, 1 out]
  n740 = global read "patternImg.vi" "New Image"() -> (w8:T5)
  n741 = call "IMAQ Dispose"("Image"=w8, "error in (no error)"=w10) -> ()  [unwired: 4 in, 1 out]
